vi "MS Auto Operation Demo.vi"() -> ()   [LabVIEW 2016]
uses:
  <vilib>/rvi/interface/nirviReadWriteControl/nirviReadWriteControl.xnode
  <vilib>/rvi/interface/nirviCloseFPGA/nirviCloseFPGA.xnode
  <vilib>/rvi/interface/nirviMethod/nirviMethod.xnode
  Subsystems/Global Variables.vi
  IRISS_FPGA_IO.vi
  <vilib>/Analysis/Matrix/Datatypes/RealMatrix.ctl
  <vilib>/Analysis/Matrix/NI_Matrix.lvlib
  Library/mjglib/var_OCTzHomeDir.vi
  Functions/EyeRobotDLL.dll
  FPGA Bitfiles/PhantomControlPI_FPGATarget_QuadCtr2_E2412E44.lvbitx
  Library/KevinLibraryAll/labview2011/kevLib2011.lvlib
  <vilib>/Math Plots/3D Math Plots/3D Scatter/3D Scatter Datatype/3D Scatter Datatype.lvclass
  <vilib>/Math Plots/3D Math Plots/3D Scatter/3D Scatter Datatype/Public/Plot Helper (Vector).vi
  <vilib>/platform/TimedLoop/XDataNode/XDataNode.xnode
  <vilib>/Platform/TimedLoop/XDataNode/nitl_modes.ctl
  <vilib>/Platform/TimedLoop/XDataNode/XDNodeRunTimeDep.lvlib
  <vilib>/Platform/TimedLoop/XDataNode/wakeup.ctl
  <vilib>/Platform/TimedLoop/XDataNode/timing_clust.ctl
  <vilib>/rvi/interface/nirviOpenFPGA/nirviOpenFPGA.xnode
  <vilib>/Utility/file.llb/Write Delimited Spreadsheet (string).vi
  <vilib>/Utility/file.llb/Write Delimited Spreadsheet (DBL).vi
  NiFpgaLv.dll
  <vilib>/Utility/error.llb/Error Cluster From Error Code.vi
  <vilib>/rvi/errors/niLvFpgaAdjustHostInterfaceError.vi
  <vilib>/FPGAPlugInAG/PXI-7833R/niLvFpga_Close_PXI-7833R.vi
  <vilib>/FPGAPlugInAG/PXI-7833R/niLvFpga_Open_PXI-7833R.vi
  <vilib>/FPGAPlugInAG/PXI-7833R/niLvFpga_Reset_PXI-7833R.vi
  <vilib>/Math Plots/3D Math Plots/3D Scatter/3D Scatter XCtrl/3D Scatter.xctl
panel:
  out "deltaRoll":sgl
  out "deltaXYZ":sgl[](array[numeric])
  out "Online Eye Model":T1
  in  "To Regulation":bool
  out "Trajectory Cluster":T2
  out "Eye Model Cluster":T4={"X Grid"=[], "Y Grid"=[], "Za_true Surf"=[], "Iris Center"=[], "Zp_true Surf"=[], "Pinv"=[[1.0, 0.0], [0.0, 1.0]], "za_true"=5.0, "za_work"=1.0, "zp_work"=-1.0, "zp_true"=-5.0}
  out "Update Mdl & Traj":bool=TRUE
  in  "Initialize":bool caption="To M/S"
  in  "Stage PID Cluster":T5={"Stage Z PID"={"Kp"=0.0005, "Kd"=0.001, "Ki"=0.0}, "Stage Y PID"={"Kp"=0.0003, "Kd"=0.01, "Ki"=0.0}, "Stage X PID"={"Kp"=0.0003, "Kd"=0.01, "Ki"=0.0}}
  in  "L1 to L4 PID Cluster":T6={"L1 PID Gains"={"Kp"=0.005, "Kd"=0.5, "Ki"=0.0005}, "L2 PID Gains"={"Kp"=0.01, "Kd"=1.0, "Ki"=0.0005}, "L3 PID Gains"={"Kp"=0.05, "Kd"=1.0, "Ki"=0.0005}, "L4 PID Gains"={"Kp"=0.1, "Kd"=1.0, "Ki"=0.0005}}
  in  "IRISS GUI":T7(tab)
  in  "Red Round Box":u32(colorbox)=16711690
  in  "Blue Round Box":u32(colorbox)=16860
  in  "Black Round Box":u32(colorbox)
  out "Vacuum Force [mmHg]  2":i32 caption="[mmHg]"
  in  "Vac Cmd [mmHg]":sgl min=0 max=600 step=50
  in  "IV Height [mmHg]":dbl=30.0 min=0.0 max=90.0 step=10.0
  in  "Irrigation":bool
  in  "Reroute Hold [sec]":dbl=10.0 caption="Hold [sec]"
  out "Next Speed":dbl=0.8 format="%#.2gx"
  out "Current Speed":dbl=0.2 format="%#_2gx"
  out "Next Depth":dbl=40.0 format="%#_g%%"
  out "Current Depth":dbl=20.0 format="%#_6g%%"
  in  "Depth Offset":dbl min=-30.0 max=70.0 step=5.0 format="%#_g%%"
  in  "Refractive Index":dbl=1.35
  in  "PO No-Fly":dbl=5.0 step=0.1 format="%#.2g"
  out "PO Cruising":dbl=5.0 format="%#.2g"
  in  "Iris Center":dbl=5.0 step=0.1 format="%#.2g"
  in  "AN Cruising":dbl=5.0 step=0.1 format="%#.2g"
  in  "AN No-Fly":dbl=5.0 step=0.1 format="%#.2g"
  in  "Iris XY Scaling":dbl[](array[numeric])=[1.0, 1.0] caption="Iris Scaling" min=0.5 max=2.0 step=0.05
  in  "Iris XY Center":dbl[](array[numeric])=[0.0, 5.0] caption="Iris Center" min=-5.0 max=5.0 step=0.25
  out "Asgn Pt Out of Bound":bool caption="Assign Pt OOB"
  out "Emergency alarm":bool
  out "Remote sender engaged":bool
  out "State changing":bool
  out "Current Run No.":u8
  out "No. of Runs":i32=5
  out "Tip out Posit":dbl[](array[numeric]) caption="Position [mm]" format="%#.3f"
  out "Tip cmd Posit":dbl[](array[numeric]) caption="Command [mm]" format="%#.3f"
  out "State Flag Array":bool[](array[boolean])
  in  "Speed Override":u16=3
  out "Timer":i32 format="%<%M:%S>t"
  in  "Assign Point [mm]":dbl[](array[numeric])=[0.0, -7.0, -6.0]
  in  "Go to Assign Pt":bool
  out "Irrigation Engaged?":bool caption="Irrigation Engaged"
  out "Robot XYZ":refnum<class "3D Plot Datatype.lvclass">[](xcontrol)
  in  "Offset":dbl[](array[numeric])
  in  "Radial Scale":dbl=0.5
  in  "Pattern":T8(ring)=enum."Centered"
  in  "Stop-and-Go":bool
  in  "SCAN_NO":string
  in  "Gen Traj":bool
  out "Trajectory OOB":bool
  out "Current System State":T9(ring)
  in  "Stage Z [mm]":dbl=100.0 min=-120.0 max=120.0 step=0.5
  in  "Stage Y [mm]":dbl=70.0 min=-120.0 max=100.0 step=0.5
  in  "Gripper":dbl
  in  "OCT Cmd Z [mm]":dbl min=-25.0 max=14.0 step=0.5
  out "Joint Out":dbl[](array[numeric])
  in  "XYZ Stage Power":bool
  in  "Arm Power":bool
  out "Robot Status Array":bool[](array[boolean])
  in  "L1 [deg]":dbl=-40.0
  in  "L2 [deg]":dbl=15.0
  in  "L3 [mm]":dbl=-5.0 step=0.1
  out "Status 2":bool[](array[boolean])
  in  "L4 [deg]":dbl=-10.0 step=0.1
  in  "Home":bool
  out "OCT Z out [mm]":dbl caption="OCT Out Z [mm]" format="%#.4f"
  in  "Tool Type":i32=6
  in  "Tool Offset [mm]":dbl=-50.68
  out "Grasp out":dbl format="%#.2g"
  in  "OCTz Home Dir":bool
  in  "OCT Z PID Gains":cluster{"Kp":dbl, "Kd":dbl, "Ki":dbl}={"Kp"=0.0003, "Kd"=0.0001, "Ki"=0.01}
  in  "Remote Control Source":u16(ring) caption="Remote Source" items=["None", "Surgical Console", "Joystick", "MJG Teleoperation", "MJG C++ Teleoperation"]
  in  "Reset Joystick":bool caption="Encoder Reset"
  out "Send Count":u64
  out "Receive Count":u64
  out "Arm ID":i32
  out "Status":bool
  in  "Stage X [mm]":dbl=30.0 min=-120.0 max=120.0 step=0.5
  out "XYZ Stage Out":dbl[](array[numeric])
  in  "Use Online Scan":bool
  out "Z Stage cmd [mm]":dbl=6.0 caption="Reference Z [mm]" min=0.0 max=12.0 step=0.5
  out "Y Stage cmd [mm]":dbl=6.0 caption="Reference Y  [mm]" min=0.0 max=12.0 step=0.5
  out "X Stage cmd [mm]":dbl=6.0 caption="Reference X [mm]" min=0.0 max=12.0 step=0.5
  in  "Process VSCAN":bool
  in  "Restart":bool
  out "Generation Error":errorcluster
  out "Model Created":bool
  out "Pressure Plots":T10(graph)
  in  "Eye No":i16=1 min=1 step=1
  in  "Reroute Transit Vacf":dbl=100.0
  in  "Z Rot Axis":dbl=1.0
  in  "Z Dist Thld":dbl[](array[numeric])=[3.0, 5.0] caption="Z Distance Threshould"
  in  "Vac Extremum":dbl[](array[numeric])=[68.0, 68.0] caption="Vacuum Extremum"
  in  "Max Limit [mmHg]":dbl=600.0 min=0.0 max=600.0 step=100.0
  out "Value [mmHg]":i8
  in  "Target IOP":sgl=20.0 min=0 max=100 step=1 format="%#_13g"
  in  "PID ON/OFF":bool
  in  "Hydration":bool
  in  "IOP PID Gains":cluster{"Kp":dbl, "Kd":dbl, "Ki":dbl, "Ts":dbl}={"Kp"=5.0, "Kd"=0.0, "Ki"=5.0, "Ts"=0.01}
  in  "Save Data":bool
  out "File Exists":bool
  out "File Path":path
  out "Elaspsed Time [s]":sgl
  in  "Data No":i16=1 min=1 step=1
  out "Pressure Reading":dbl[](array[numeric]) caption="IOP Output [mmHg]"
  in  "Total Time":i16=90 min=1 step=1
  in  "Min PC Gap":dbl=0.1 caption="Min PC Gap [mm]" min=0.0 max=10.0 step=0.1 format="%#.3g"
  in  "Min AC Gap":dbl=0.1 caption="Min AC Gap [mm]" min=0.0 max=10.0 step=0.1 format="%#.3g"
  out "Scaling":dbl[](array[numeric])=[1.0, 1.0, 1.0] caption="S" min=0.5 max=1.5 step=0.05 format="%#_3g"
  in  "Joint Limits":dbl[][](array[numeric])=[[-68.0, -4.0], [-26.0, 52.0], [-40.0, 23.0], [-180.0, 180.0]] format="%#.3g"
  out "First Trk Pt":dbl[](array[numeric]) format="%#.3g"
  out "Error(s) Out on Program End":errorcluster
  out "L4 Waveform Graph":dbl[](graph)
  out "L3 Waveform Graph":dbl[](graph)
  out "L2 Waveform Graph":dbl[](graph)
  out "L1 Waveform Graph":dbl[](graph)
  in  "Aiming Pt":dbl[](array[numeric])=[-40.0, 11.0, 2.0, 0.0] format="%#.3g"
  in  "Engage Pt":dbl[](array[numeric])=[-40.0, 11.0, 2.0, 0.0] format="%#.3g"
  in  "Rotation":dbl[](array[numeric])=[0.0, 0.0, 0.0] caption="R [deg]" min=-15.0 max=15.0 step=0.5 format="%#_3g"
  out "Translation":dbl[](array[numeric]) caption="T [mm]" min=-3.0 max=3.0 step=0.1 format="%#_3g"
  in  "Inc Ctrl":dbl[](array[numeric])=[0.1, 0.05, 0.05] caption="Increment Control"
  in  "Depth Ctrl Array\n(% Thickness)":dbl[](array[numeric])=[40.0, 60.0, 80.0] min=10.0 max=90.0 step=5.0 format="%#_g%%"
  in  "Load Traj":bool caption="To M/S"
  in  "MS/Auto":bool
  in  "Retract":bool caption="To M/S"
  in  "Stop Accurus":bool caption="To M/S"
  in  "L3 Go Home":bool caption="To M/S"
  in  "Track":bool caption="To M/S"
  in  "Insert":bool caption="To M/S"
  in  "Program Stop":bool
  # "M/S\n\nAuto"
  # "Tool Tip Location"
  # "Tracking Planning"
  # "RCM"
  # "X\nY\nZ"
  # "X\nY\nZ"
  # "Tool"
  # "Trajectory"
  # "System Progress"
  # "Assign Point Rerouting"
  # "Trajectory Generation"
  # "X\nY\nZ"
  # "X Offset"
  # "Y Offset"
  # "Homing finished"
  # "Z Offset"
  # "M/S initialization finished"
  # "Tool Cruising Boundaries"
  # "XY-plane"
  # "Trajecoty loading finished"
  # "Aiming finished"
  # "Tool engaged"
  # "Z-axis"
  # "Tracking initialization finished"
  # "In Tracking"
  # "Bausch Lomb"
  # "Rerouting finished"
  # "X\nY"
  # "X\nY"
  # "In regulation"
  # "Homing"
  # "Robot Control"
  # "Joint Definition"
  # "Arm"
  # "Tool"
  # "Stage"
  # "Joint M/S Cmd"
  # "Robot Status"
  # "ROBOT_HARDWARE_NOT_PRESENT"
  # "ROBOT_HARDWARE_NOT_FOUND_ALL_DRIVES"
  # "ROBOT_HARDWARE_SENSOR_FAULT"
  # "ROBOT_NOT_RUNNING"
  # "ROBOT_COMMUNICATION_ERROR"
  # "OCT Control"
  # "ROBOT_KINEMATICS_NO_SOLUTION"
  # "ROBOT_KINEMATICS_INSERTION_LENGTH_TOO_SMALL"
  # "ROBOT_COMMAND_BEYOND_JOINT_RANGE"
  # "ROBOT_COMMAND_TOO_LARGE"
  # "XYZ Stage Control"
  # "Eye Model Creation"
  # "Irrigation and Aspiration"
  # "IOP Control"
  # "Data Saving"
  # "Irrigation"
  # "Aspiration"
  # "ACh"
  # "Vitreous"
  # "Rotation & Vacuum Force Scheduling"
  # "Joint Motion & Control"
  # "Space Deform Parameters"
  # "Depth Ctrl"
  # "S"
  # "R"
  # "[deg]"
  # "T"
  # "[mm]"
  # "First Track Point"
  # "AC & PC Gap"
  # "X1"
  # "[mm]"
  # "Y"
  # "[mm]"
  # "Z"
  # "[mm]"
  # "L4"
  # "[deg]"
  # "Joint Limits"
  # "Error Message"
  # "Incision"
  # "Min."
  # "Max."
  # "L1"
  # "[deg]"
  # "L1"
  # "L2"
  # "L2"
  # "[deg]"
  # "L3"
  # "[mm]"
  # "L3"
  # "L4"
  # "[deg]"
  # "L4"
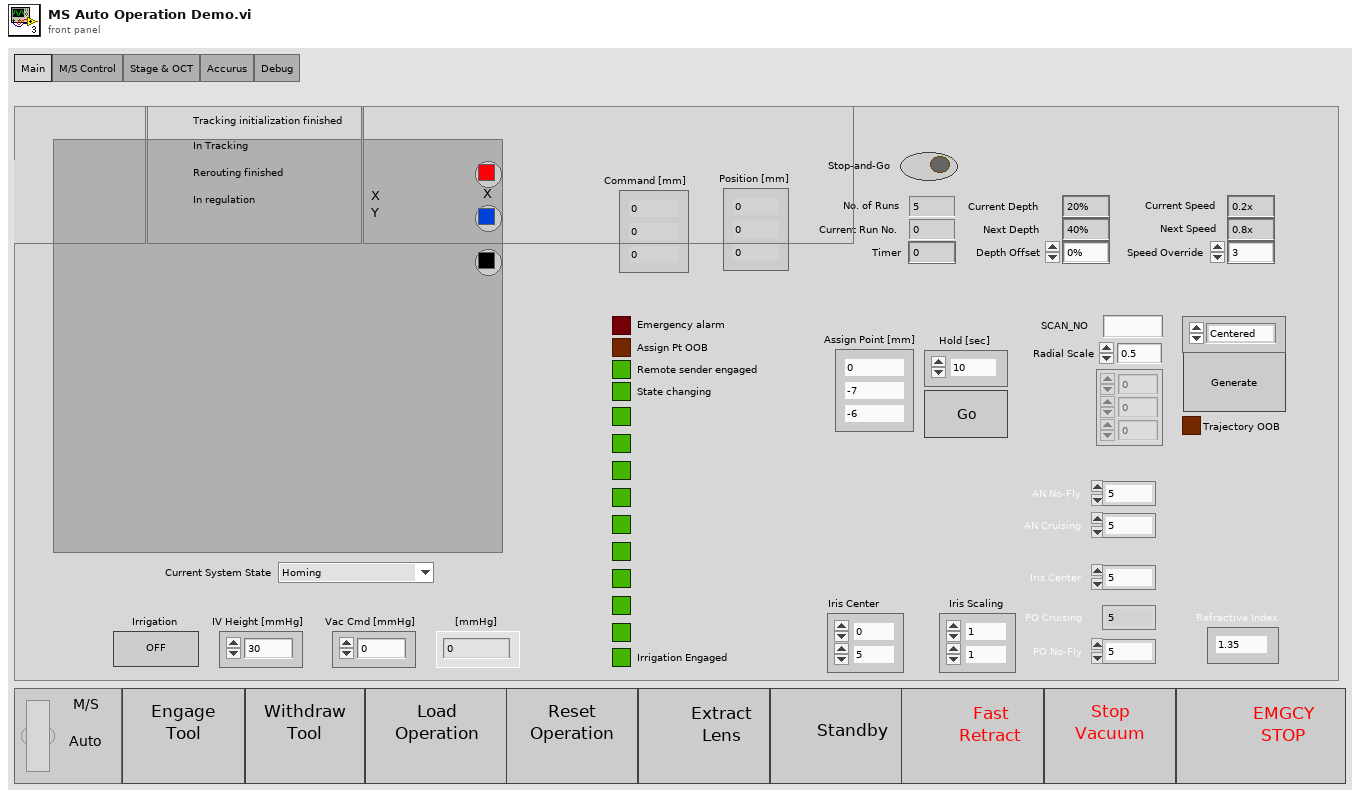
[diagram p1: front panel]
types:
  T1 = cluster{"za_true":dbl, "za_work":dbl, "zi":dbl, "zp_work":dbl, "zp_true":dbl, "Iris XY Center":dbl[], "Iris XY Scaling":dbl[]}
  T2 = cluster{"Traj Px Array":dbl[], "Traj Py Array":dbl[], "Traj Pz Array":dbl[], "Speed Array":dbl[], "Depth Array":dbl[]}
  T3 = typedef "NI_Matrix.lvlib/RealMatrix.ctl" = dbl[][]
  T4 = cluster{"X Grid":dbl[], "Y Grid":dbl[], "Za_true Surf":dbl[][], "Iris Center":dbl[], "Zp_true Surf":dbl[][], "Pinv":T3, "za_true":dbl, "za_work":dbl, "zp_work":dbl, "zp_true":dbl}
  T5 = cluster{"Stage Z PID":cluster{"Kp":dbl, "Kd":dbl, "Ki":dbl}, "Stage Y PID":cluster{"Kp":dbl, "Kd":dbl, "Ki":dbl}, "Stage X PID":cluster{"Kp":dbl, "Kd":dbl, "Ki":dbl}}
  T6 = cluster{"L1 PID Gains":cluster{"Kp":dbl, "Kd":dbl, "Ki":dbl}, "L2 PID Gains":cluster{"Kp":dbl, "Kd":dbl, "Ki":dbl}, "L3 PID Gains":cluster{"Kp":dbl, "Kd":dbl, "Ki":dbl}, "L4 PID Gains":cluster{"Kp":dbl, "Kd":dbl, "Ki":dbl}}
  T7 = enum32{"Main", "M/S Control", "Stage & OCT", "Accurus", "Debug"}
  T8 = enum16{"Entry Site", "Centered", "Insertion", "Extraction", "Reverse Entry Site", "Reverse Centered"}
  T9 = enum16{"Homing", "M/S Initialization", "M/S Operation", "Aiming", "Engaging", "Trajectory Loading", "Tracking Initialization", "Tracking", "Rerouting", "Regulation"}
  T10 = cluster{"Pressure Reading[0]":dbl, "Pressure Reading[1]":dbl, "Pressure Reading[2]":dbl, "Pressure Reading[3]":dbl, "Pressure Reading[4]":dbl, "Pressure Reading[5]":dbl, "Pressure Reading[6]":dbl, "Pressure Reading[7]":dbl, "Pressure Reading[8]":dbl}
  T11 = cluster{"Prev L1 to L4 Posit":dbl[], "Prev Stage Posit":dbl[], "Prev OCT Z Posit":dbl}
  T12 = typedef "XDNodeRunTimeDep.lvlib/timing_clust.ctl" = cluster{"Expected End [f-1]":u64, "Actual End [f-1]":u64, "Finished Late? [f-1]":bool, "Expected End [i-1]":u64, "Actual End [i-1]":u64, "Finished Late? [i-1]":bool, "Expected Start [i]":u64, "Actual Start [i]":u64, "Expected Start [f]":u64, "Actual Start [f]":u64, "Source Name":string, "Structure Name":string, "Period":i64, "Deadline":i64, "Offset":i64, "Start":i64, "Priority":i32, "Timeout":i32, "Mode":T13, "Wakeup Reason":T14, "Error":errorcluster, "Source Type":string, "Secondary Source Type":string, "Global End Time":u64, "Global Start Time":u64, "Frame Duration":u64, "Iteration Duration":u64, "Assigned CPU":i32, "I/O Scan Engine Mode":u32}
  T13 = typedef "XDNodeRunTimeDep.lvlib/nitl_modes.ctl" = enum32{"No Change", "Process missed periods, maintain original phase", "Discard missed periods, maintain original phase", "Process missed periods, ignore original phase", "Discard missed periods, ignore original phase"}
  T14 = typedef "XDNodeRunTimeDep.lvlib/wakeup.ctl" = enum32{"Normal", "Aborted", "Asynchronous wakeup", "Timing source error", "Timed loop error", "Timeout"}
  T15 = cluster{"L1 to L4 PID Cluster":cluster{"L1 PID Gains":cluster{"Kp":dbl, "Kd":dbl, "Ki":dbl}, "L2 PID Gains":cluster{"Kp":dbl, "Kd":dbl, "Ki":dbl}, "L3 PID Gains":cluster{"Kp":dbl, "Kd":dbl, "Ki":dbl}, "L4 PID Gains":cluster{"Kp":dbl, "Kd":dbl, "Ki":dbl}}, "Stage PID Cluster":cluster{"Stage Z PID":cluster{"Kp":dbl, "Kd":dbl, "Ki":dbl}, "Stage Y PID":cluster{"Kp":dbl, "Kd":dbl, "Ki":dbl}, "Stage X PID":cluster{"Kp":dbl, "Kd":dbl, "Ki":dbl}}, "OCT Z PID Gains":cluster{"Kp":dbl, "Kd":dbl, "Ki":dbl}}
  T16 = enum8{"Enabled", "Disabled", "Disabled and Grayed Out"}
  T17 = cluster{"IOP Output [mmHg][0]":dbl, "IOP Output [mmHg][1]":dbl, "IOP Output [mmHg][2]":dbl, "IOP Output [mmHg][3]":dbl, "IOP Output [mmHg][4]":dbl, "IOP Output [mmHg][5]":dbl, "IOP Output [mmHg][6]":dbl, "IOP Output [mmHg][7]":dbl, "IOP Output [mmHg][8]":dbl}
  T18 = cluster{"Last L1 to L4 Posit":dbl[], "Last Stage Posit":dbl[], "Last OCT Z Posit":dbl}
  T19 = cluster{"za_true_0":dbl, "za_work_0":dbl, "zp_work_0":dbl, "zp_true_0":dbl, "IrisCenter_0":dbl[]}
  T20 = cluster{"X Grid":dbl[], "Y Grid":dbl[], "Za_true Surf":dbl[][], "Iris Center":dbl[], "Zp_true Surf":dbl[][], "Real Matrix":T3, "za_true":dbl, "za_work":dbl, "zp_work":dbl, "zp_true":dbl}
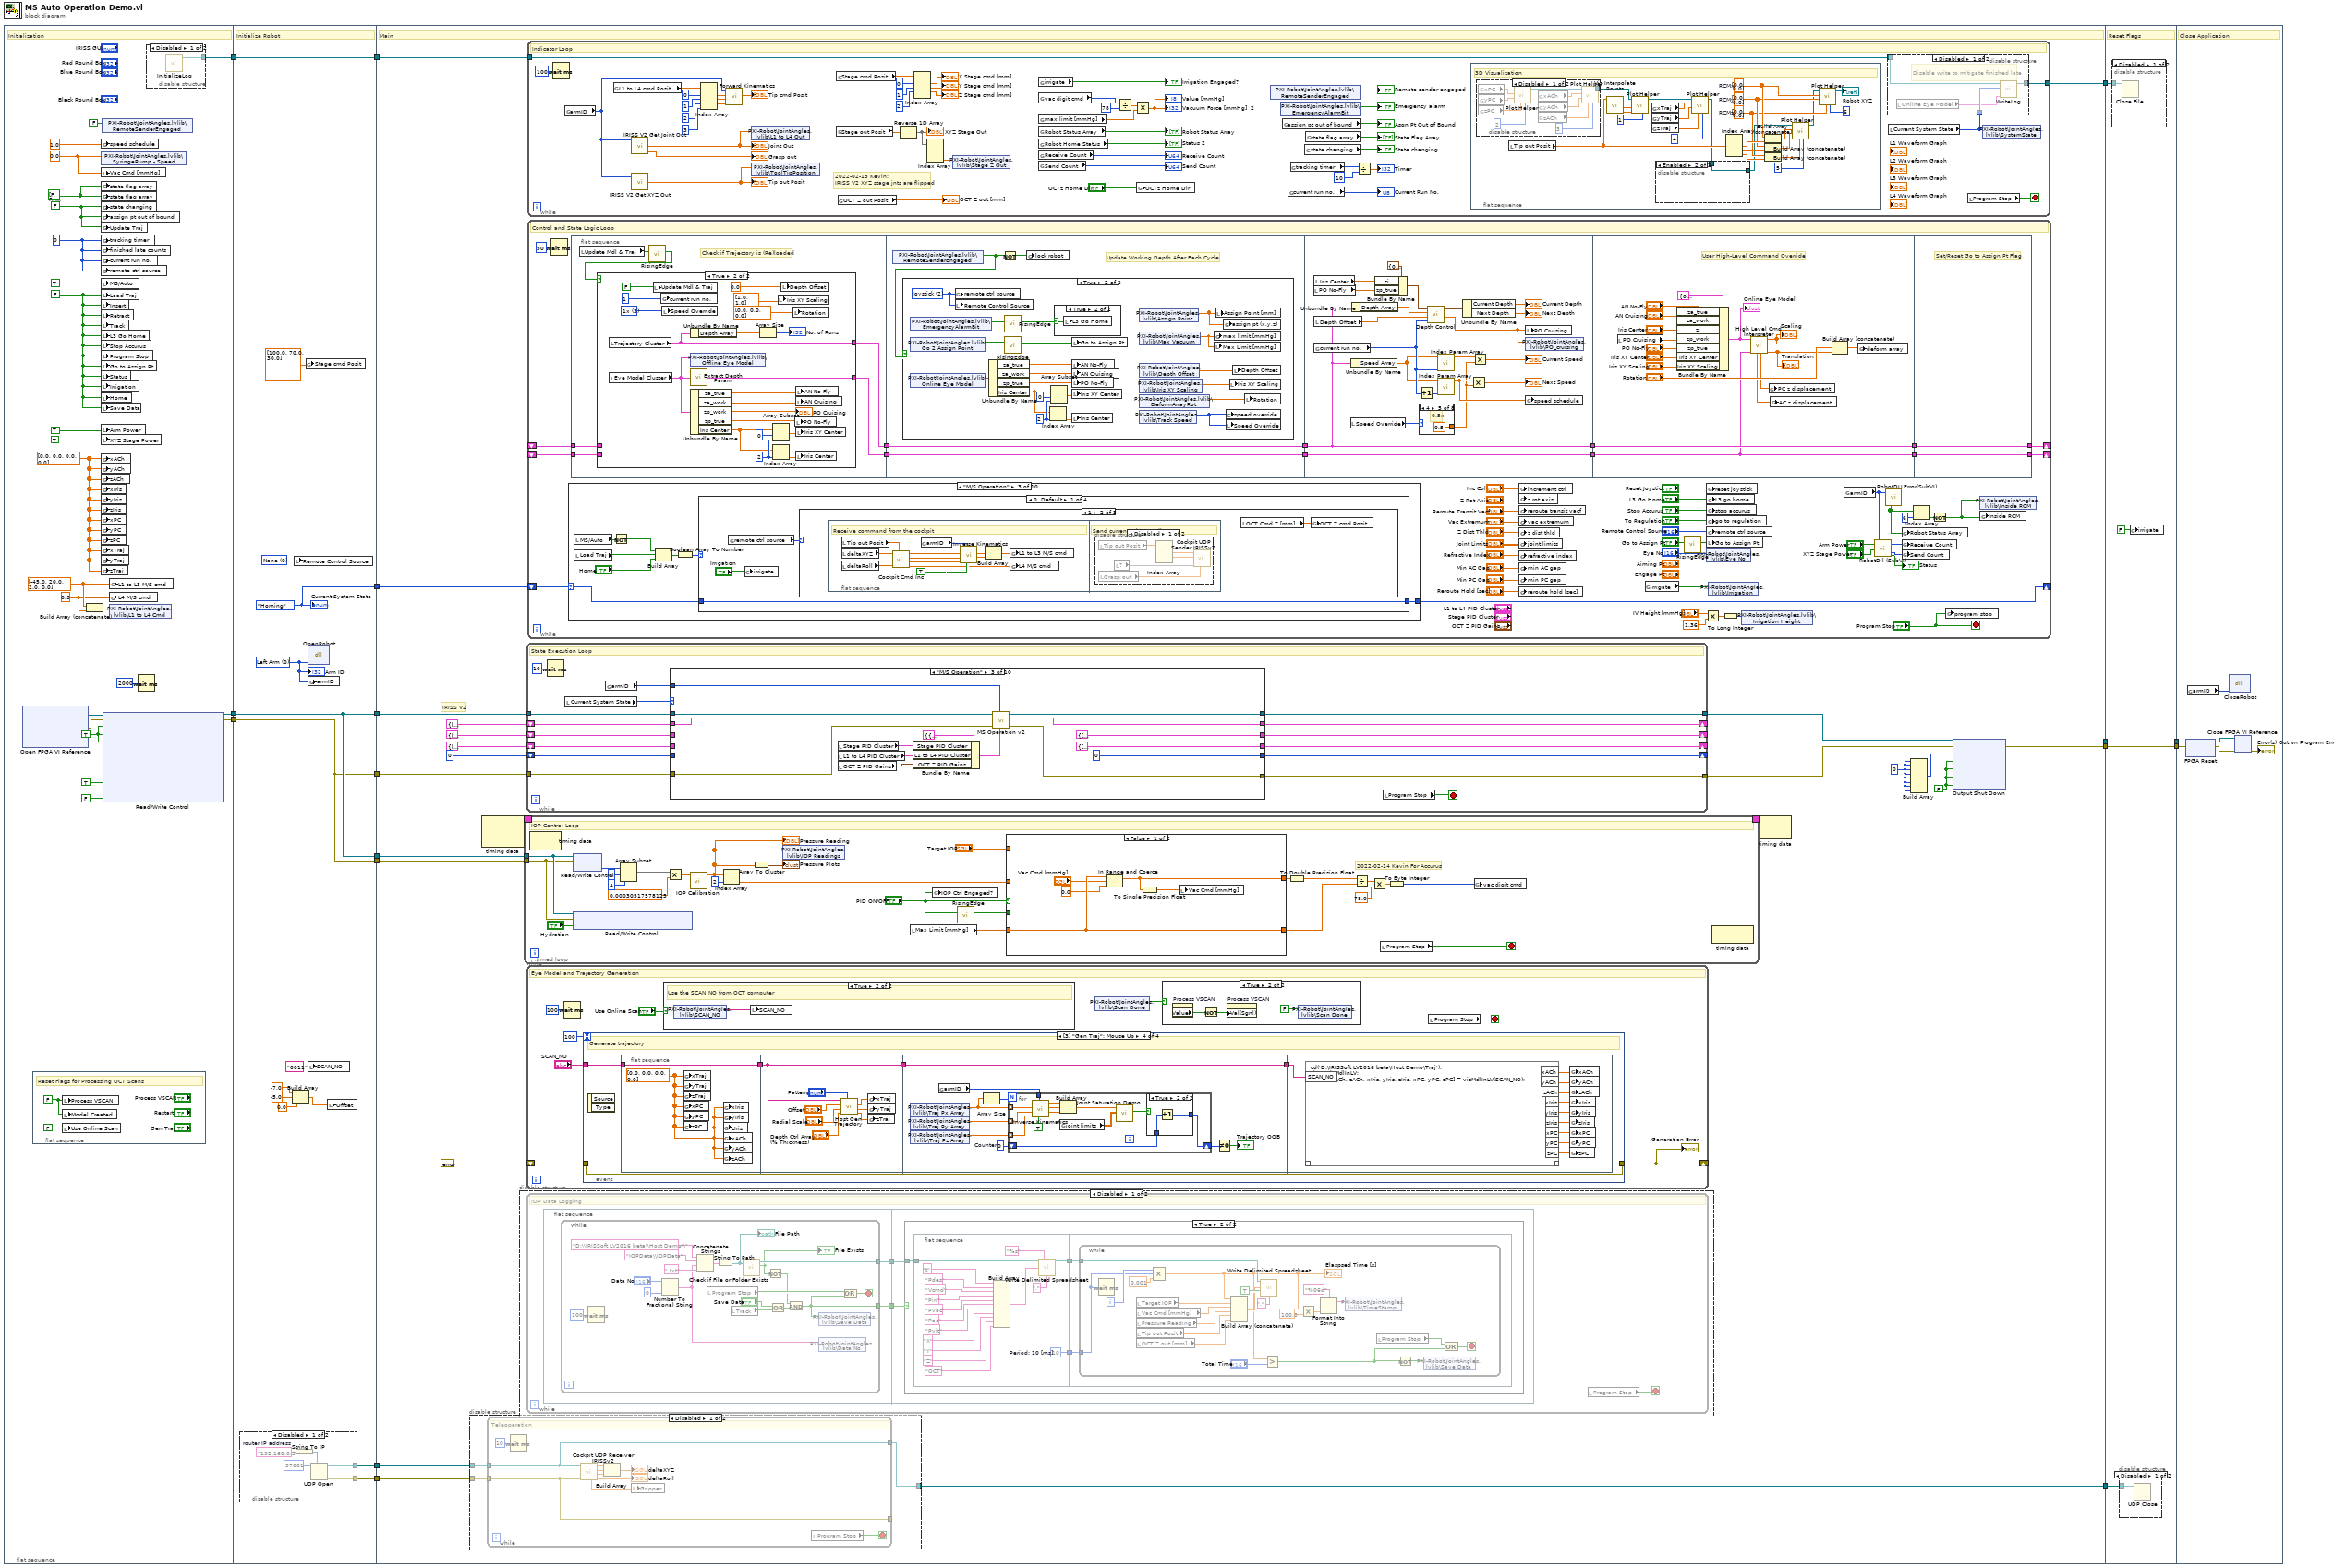
[diagram p0: block diagram]
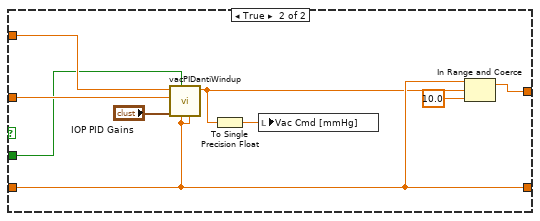
[diagram p7: hidden frame]
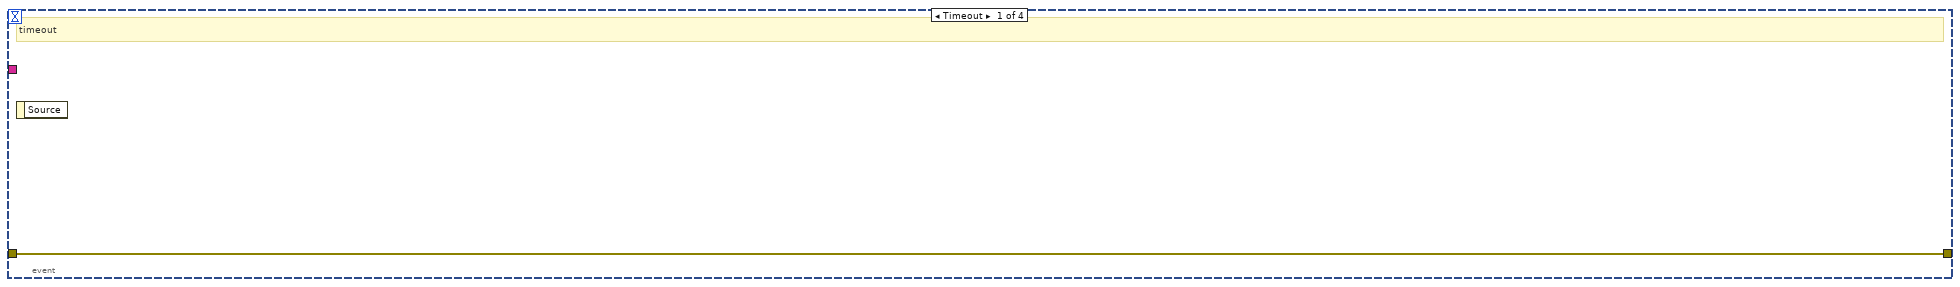
[diagram p10: hidden frame]
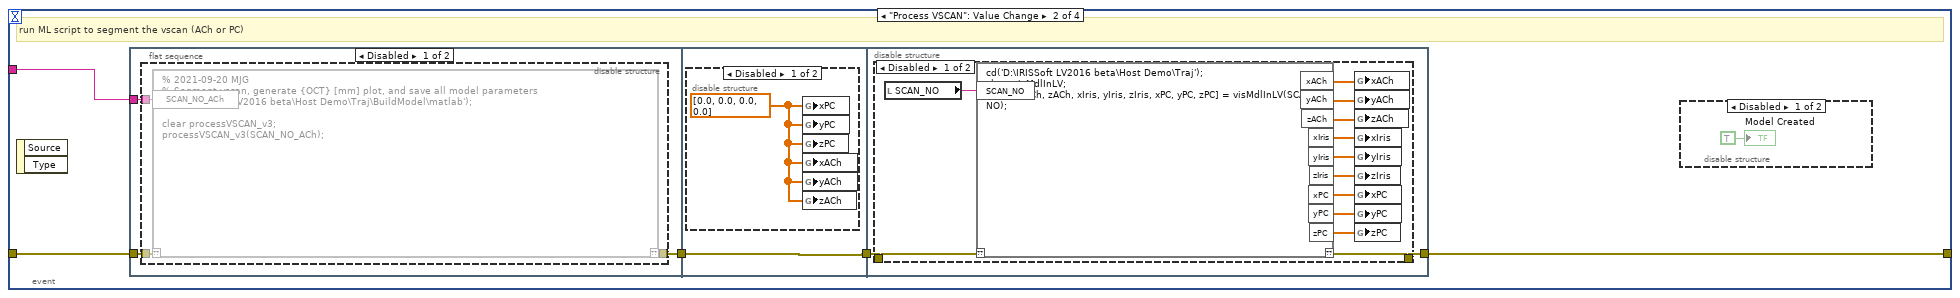
[diagram p11: hidden frame]
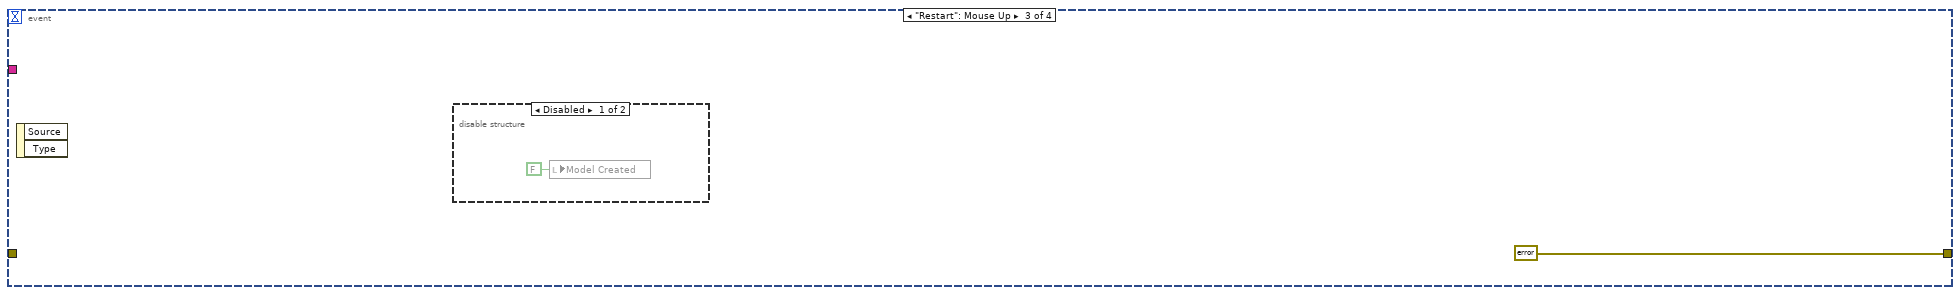
[diagram p16: hidden frame]
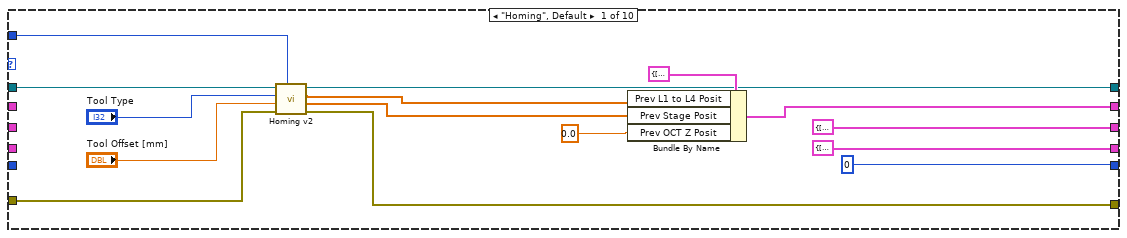
[diagram p19: hidden frame]
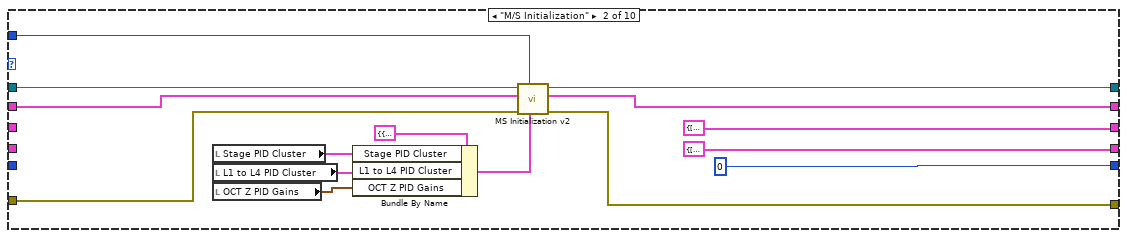
[diagram p20: hidden frame]
diagram:
  n1 = flat-sequence {
    tunnel: [w39] -> w9
    tunnel: [w27] -> w5
    tunnel: [w26] -> w4
    tunnel: [w54] -> w12
    tunnel: [w55] -> w11
    tunnel: [w53] -> w10
    tunnel: w9 -> [w57]
    tunnel: [w57] -> w8
    tunnel: [w55] -> w7
    tunnel: [w54] -> w6
    tunnel: w5 -> [w55]
    tunnel: w4 -> [w54]
    tunnel: [w52] -> w3
    tunnel: [w51] -> w2
    tunnel: w12 -> [w83]
    tunnel: w11 -> [w80]
    tunnel: w10 -> [w86]
    tunnel: [w81] -> w17
    tunnel: [w82] -> w16
    tunnel: w8 -> [w85]
    tunnel: [w84] -> w15
    tunnel: w7 -> [w70]
    tunnel: w6 -> [w69]
    tunnel: w3 -> [w65]
    tunnel: w2 -> [w64]
    tunnel: [w63] -> w1
    tunnel: w17 -> [w1060]
    tunnel: w16 -> [w1061]
    tunnel: w15 -> [w1062]
    tunnel: [w1061] -> w14
    tunnel: [w1060] -> w13
    tunnel: w1 -> [w1058]
    tunnel: w14 -> [w1070]
    tunnel: w13 -> [w1069]
    frame #0 {
      w28 = TRUE ("Conn0/DIO13 Button 2")
      w24 = dbl[] [0.0, 0.0, 0.0, 0.0] ("First Trk Pt 2")
      w34 = 0.0 ("L4 M/S cmd")
      w35 = dbl[] [-45.0, 20.0, 2.0, 0.0] ("First Trk Pt 2")
      w38 = 0.0 ("SyringePump - Speed")
      w23 = 0 ("finished late counts")
      w37 = bool[] [FALSE, FALSE, FALSE, FALSE, FALSE, FALSE, FALSE, FALSE, FALSE] ("state flag array")
      w32 = FALSE ("state changing")
      w25 = FALSE ("program stop")
      # "Initialization"
      n2 = xnode "Open FPGA VI Reference"() -> ("FPGA VI Reference Out"=w22:refnum<k20>, "error out"=w21:errorcluster)  [unwired: 2 in]
      n3 = flat-sequence {
        frame #0 {
          w41 = FALSE ("ACh Processed")
          # "Reset Flags for Processing OCT Scans"
          n4 = local write "Process VSCAN"(w41) -> ()
          n5 = local write "Model Created"(w41) -> ()
          n6 = local write "Use Online Scan"(FALSE ("Use Online Scan")) -> ()
        }
      }
      n7 = Build Array (concatenate)(w35, w34) -> (w33:dbl[])
      n8 = global write "Global Variables.vi" "speed schedule"(1.0 ("speed schedule")) -> ()
      n9 = shared-variable "PXI-Robot\\JointAngles.lvlib\\SyringePump - Speed"(w38) -> ()  [unwired: 1 in, 1 out]
      n10 = local write "Vac Cmd [mmHg]"(w38) -> ()
      n11 = global write "Global Variables.vi" "state flag array"(w37) -> ()
      n12 = global write "Global Variables.vi" "state flag array"(w37) -> ()
      n13 = global write "Global Variables.vi" "state changing"(w32) -> ()
      n14 = global write "Global Variables.vi" "assign pt out of bound"(w32) -> ()
      n15 = global write "Global Variables.vi" "Update Traj"(w32) -> ()
      n16 = global write "Global Variables.vi" "tracking timer"(w23) -> ()
      n17 = global write "Global Variables.vi" "finished late counts"(w23) -> ()
      n18 = global write "Global Variables.vi" "current run no."(w23) -> ()
      n19 = global write "Global Variables.vi" "remote ctrl source"(w23) -> ()
      n20 = local write "MS/Auto"(TRUE ("MS/Auto")) -> ()
      n21 = local write "Load Traj"(w25) -> ()
      n22 = local write "Insert"(w25) -> ()
      n23 = local write "Retract"(w25) -> ()
      n24 = local write "Track"(w25) -> ()
      n25 = local write "L3 Go Home"(w25) -> ()
      n26 = local write "Stop Accurus"(w25) -> ()
      n27 = local write "Program Stop"(w25) -> ()
      n28 = local write "Go to Assign Pt"(w25) -> ()
      n29 = local write "Status"(w25) -> ()
      n30 = local write "Irrigation"(w25) -> ()
      n31 = local write "Home"(w25) -> ()
      n32 = local write "Save Data"(w25) -> ()
      n33 = local write "Arm Power"(TRUE ("Arm ON/OFF")) -> ()
      n34 = local write "XYZ Stage Power"(TRUE ("Arm ON/OFF")) -> ()
      n35 = global write "Global Variables.vi" "xACh"(w24) -> ()
      n36 = global write "Global Variables.vi" "yACh"(w24) -> ()
      n37 = global write "Global Variables.vi" "zACh"(w24) -> ()
      n38 = global write "Global Variables.vi" "xIris"(w24) -> ()
      n39 = global write "Global Variables.vi" "yIris"(w24) -> ()
      n40 = global write "Global Variables.vi" "zIris"(w24) -> ()
      n41 = global write "Global Variables.vi" "xPC"(w24) -> ()
      n42 = global write "Global Variables.vi" "yPC"(w24) -> ()
      n43 = global write "Global Variables.vi" "zPC"(w24) -> ()
      n44 = global write "Global Variables.vi" "xTraj"(w24) -> ()
      n45 = global write "Global Variables.vi" "yTraj"(w24) -> ()
      n46 = global write "Global Variables.vi" "zTraj"(w24) -> ()
      n47 = shared-variable "PXI-Robot\\JointAngles.lvlib\\RemoteSenderEngaged"(FALSE ("RemoteSenderEngaged")) -> ()  [unwired: 1 in, 1 out]
      n48 = xnode "Read/Write Control"("FPGA VI Reference In"=w22, "error in"=w21, "Conn0/DIO12 Button 1"=w28, "Conn0/DIO13 Button 2"=w28, "Conn0/DIO15 Button 4"=w28, "Reset 14"=TRUE, "Hydration On/Off (Connector2/DIO28)"=FALSE) -> ("FPGA VI Reference Out"=w27:refnum<k20>, "error out"=w26:errorcluster)  [unwired: 3 in, 2 out]
      n49 = global write "Global Variables.vi" "L1 to L3 M/S cmd"(w35) -> ()
      n50 = global write "Global Variables.vi" "L4 M/S cmd"(w34) -> ()
      n51 = shared-variable "PXI-Robot\\JointAngles.lvlib\\L1 to L4 Cmd"(w33) -> ()  [unwired: 1 in, 1 out]
      n52 = Wait (ms)(milliseconds to wait=u32 2000) -> ()  [unwired: 1 out]
      n53 = disable-structure shown="Disabled" {
        disable-tunnel: [w43 _] -> w39
        frame Disabled {
          n54 = call "InitializeLog.vi"() -> ("Byte Stream File out"=w43:refnum<file>)  [unwired: 11 in]
        }
        frame Enabled {
        }
      }
    }
    frame #1 {
      w49 = u16 0 items=["None", "Surgical Console", "Joystick", "MJG Teleoperation", "MJG C++ Teleoperation"] ("Remote Control Source 2")
      w53 = T9."Homing" ("Current State")
      w56 = 0 items=["Left Arm", "Right Arm"] ("Left or Right Arm")
      # "Initialize Robot"
      n55 = disable-structure shown="Disabled" {
        disable-tunnel: [w59 _] -> w52
        disable-tunnel: [w58 _] -> w51
        frame Disabled {
          w61 = "192.168.0.3"  # router IP address
          n56 = String To IP(1:w61) -> (0:w60:u32)
          n57 = UDP Open(7:w60, 11:u16 37001 ("port")) -> (port=w59:refnum<k16>, 0:w58:errorcluster)  [unwired: 3 in, 1 out]
        }
        frame Enabled {
        }
      }
      n58 = Build Array(-7.0 ("element"), -5.0 ("element"), 0.0 ("element")) -> (w48:dbl[])
      n59 = local write "Remote Control Source"(w49) -> ()
      n60 = global write "Global Variables.vi" "Stage cmd Posit"(dbl[] [100.0, 70.0, 30.0] ("Stage cmd Posit")) -> ()
      n61 = dll-call lib="D:/Kevin/IRISS V2 dev/Host Demo/Functions/EyeRobotDLL.dll" fn="OpenRobot" label="Open"("id"=w56) -> ()  [unwired: 5 in, 2 out]
      n62 = global write "Global Variables.vi" "armID"(w56) -> ()
      n63 = local write "SCAN_NO"("0011" ("SCAN_NO")) -> ()
      n64 = local write "Offset"(w48) -> ()
      "Arm ID" <- w56
      "Current System State" <- w53
    }
    frame #2 {
      w68 = FALSE
      w66 = i16 0 ("element")
      # "IRISS V2"
      # "Main"
      n65 = disable-structure shown="Disabled" {
        disable-tunnel: w65 -> [w158 _]
        disable-tunnel: w64 -> [w157 _]
        disable-tunnel: [w156 _] -> w63
        frame Disabled {
          n66 = while {
            tunnel: w158 -> [w165]
            tunnel: w157 -> [w164]
            tunnel: [w165] -> w156
            tunnel: [w164] -> _
            stop <- w163 stop-if-true
            # "Teleoperation"
            n67 = Wait (ms)(milliseconds to wait=u32 10) -> ()  [unwired: 1 out]
            n68 = call "Cockpit UDP Receiver IRISSv2.vi"("error in"=w164, "port"=w165) -> ("deltaRoll"=→"deltaRoll":sgl, "deltaZ"=w166:sgl, "deltaY"=w167:sgl, "deltaX"=w168:sgl, "gripper"=w160:sgl)  [unwired: 5 in]
            n69 = Build Array(w168, w167, w166) -> (→"deltaXYZ":sgl[])
            n70 = local write "Gripper"(w160) -> ()
            n71 = local read "Program Stop"() -> (w163:bool)
          }
        }
        frame Enabled {
        }
      }
      n72 = node-c288() -> (w72:T12)  [unwired: 2 in]
      n73 = disable-structure shown="Disabled" {
        frame Disabled {
          n74 = while {
            stop <- w87 stop-if-true
            # "IOP Data Logging"
            n75 = flat-sequence {
              tunnel: [w90] -> w89
              tunnel: [w91] -> w88
              tunnel: w89 -> [w111]
              tunnel: w88 -> [w110]
              frame #0 {
                n76 = while {
                  tunnel: [w108] -> w91
                  tunnel: [w92] -> w90
                  stop <- w109 stop-if-true
                  n77 = Wait (ms)(milliseconds to wait=u32 100) -> ()  [unwired: 1 out]
                  n78 = Number To Fractional String(number="Data No", precision (6)=i16 0) -> (F-format string=w98:string)  [unwired: 2 in]
                  n79 = Concatenate Strings("D:\\IRISSoft LV2016 beta\\Host Demo\\", "IOPData\\IOPData", w98, ".txt" ("string")) -> (w104:string)
                  n80 = local read "Program Stop"() -> (w105:bool)
                  n81 = String To Path(string=w104) -> (path=w100:path)
                  "File Path" <- w100
                  n82 = local read "Track"() -> (w95:bool)
                  n83 = call <vilib>:"Check if File or Folder Exists.vi"("path"=w100) -> ("file or folder exists?"=w106:bool, "dup path"=w108:path)  [unwired: 8 in, 1 out]
                  "File Exists" <- w106
                  n84 = Not(x=w106) -> (.not. x?=w94:bool)
                  n85 = Or(x="Save Data", y=w95) -> (x .or. y?=w93:bool)
                  n86 = Compound Arithmetic op=AND(w94, w93) -> (w92:bool)
                  n87 = shared-variable "PXI-Robot\\JointAngles.lvlib\\Save Data"(w92) -> ()  [unwired: 1 in, 1 out]
                  n88 = shared-variable "PXI-Robot\\JointAngles.lvlib\\Data No"(w98) -> ()  [unwired: 1 in, 1 out]
                  n89 = Compound Arithmetic op=OR(w105, w92) -> (w109:bool)
                }
              }
              frame #1 {
                n90 = case shown="True" w111 {
                  tunnel: w110 -> [_ w114]
                  frame False {
                  }
                  frame True {
                    n91 = flat-sequence {
                      tunnel: w114 -> [w125]
                      tunnel: [w123] -> w113
                      tunnel: [w119] -> w112
                      tunnel: w113 -> [w133]
                      tunnel: w112 -> [w132]
                      frame #0 {
                        w119 = 10  # Period: 10 [ms]
                        n92 = Build Array("t" ("delimiter (\\t)"), "Pdes" ("delimiter (\\t)"), "Vcmd" ("delimiter (\\t)"), "Pirr" ("delimiter (\\t)"), "Pvac" ("delimiter (\\t)"), "Pac" ("delimiter (\\t)"), "Pvit" ("delimiter (\\t)"), "X" ("delimiter (\\t)"), "Y" ("delimiter (\\t)"), "Z" ("delimiter (\\t)"), "OCT" ("delimiter (\\t)")) -> (w122:string[])
                        n93 = call-poly <vilib>:"Write Delimited Spreadsheet.vi"("file path (dialog if empty)"=w125, "format (%s)"="%s", "1D data"=w122, "delimiter (\\t)"="," ("delimiter (\\t)")) -> ("new file path (Not A Path if cancelled)"=w123:path)  [unwired: 10 in, 1 out]
                      }
                      frame #1 {
                        n94 = while {
                          tunnel: w133 -> [w152]
                          tunnel: w132 -> [w138]
                          i -> [w153]
                          stop <- w155 stop-if-true
                          n95 = Wait (ms)(milliseconds to wait=w138) -> ()  [unwired: 1 out]
                          n96 = local read "Target IOP"() -> (w148:sgl)
                          n97 = local read "Vac Cmd [mmHg]"() -> (w147:sgl)
                          n98 = local read "Pressure Reading"() -> (w146:dbl[])
                          n99 = local read "Tip out Posit"() -> (w143:dbl[])
                          n100 = local read "OCT Z out [mm]"() -> (w144:dbl)
                          n101 = Compound Arithmetic op=MULTIPLY(w153, w138, 0.001 ("y")) -> (w135:dbl)
                          "Elaspsed Time [s]" <- w135
                          n102 = Build Array (concatenate)(w135, w148, w147, w146, w143, w144) -> (w150:dbl[])
                          n103 = call-poly <vilib>:"Write Delimited Spreadsheet.vi"("file path (dialog if empty)"=w152, "1D data"=w150, "append to file? (new file:F)"=TRUE, "delimiter (\\t)"="," ("delimiter (\\t)")) -> ()  [unwired: 10 in, 2 out]
                          n104 = Greater?(x=w135, y="Total Time") -> (0:w136:bool)
                          n105 = Multiply(x=w135, y=100.0) -> (x*y=w140:dbl)
                          n106 = Format Into String(format string="%06d", w140) -> (resulting string=w141:string)  [unwired: 2 in, 1 out]
                          n107 = shared-variable "PXI-Robot\\JointAngles.lvlib\\TimeStamp"(w141) -> ()  [unwired: 1 in, 1 out]
                          n108 = local read "Program Stop"() -> (w145:bool)
                          n109 = Not(x=w136) -> (.not. x?=w137:bool)
                          n110 = shared-variable "PXI-Robot\\JointAngles.lvlib\\Save Data"(w137) -> ()  [unwired: 1 in, 1 out]
                          n111 = Compound Arithmetic op=OR(w145, w136) -> (w155:bool)
                        }
                      }
                    }
                  }
                }
              }
            }
            n112 = local read "Program Stop"() -> (w87:bool)
          }
        }
        frame Enabled {
        }
      }
      n113 = timed-loop {
        timing: w72 -> [_]
        timing-out: [_] -> w71
        tunnel: w70 -> [w193]
        tunnel: w69 -> [w192]
        stop <- w188 stop-if-true
        # "2022-02-14 Kevin For Accurus"
        # "IOP Control Loop"
        n114 = node-c288() -> ()  [unwired: 1 in, 1 out]
        n115 = xnode "Read/Write Control"("FPGA VI Reference In"=w193, "error in"=w192) -> ("AI"=w187:i16[])  [unwired: 2 out]
        n116 = xnode "Read/Write Control"("FPGA VI Reference In"=w193, "error in"=w192, "Hydration On/Off (Connector2/DIO28)"="Hydration") -> ()  [unwired: 2 out]
        n117 = Array Subset(array=w187, index=0, length=4) -> (w184:i16[])
        n118 = Multiply(x=w184, y=0.00030517578125) -> (x*y=w182:dbl[])
        n119 = call "IOP Calibration.vi"("IOP Input [V]"=w182) -> ("IOP Output [mmHg]"=w172:dbl[])  [unwired: 10 in]
        "Pressure Reading" <- w172
        n120 = Index Array(array=w172, index=2) -> (element=w190:dbl)
        n121 = Array To Cluster(array=w172) -> (cluster=→"Pressure Plots":T17)
        n122 = shared-variable "PXI-Robot\\JointAngles.lvlib\\IOP Readings"(w172) -> ()  [unwired: 1 in, 1 out]
        n123 = local read "Max Limit [mmHg]"() -> (w189:dbl)
        n124 = global write "Global Variables.vi" "IOP Ctrl Engaged?"("PID ON/OFF") -> ()
        n125 = call "RisingEdge.vi"("Signal In"="PID ON/OFF") -> ("Rising Edge"=w179:bool)  [unwired: 10 in]
        n126 = case shown="False" "PID ON/OFF" {
          tunnel: "Target IOP" -> [_ w207]
          tunnel: w190 -> [_ w206]
          tunnel: w189 -> [w198 w201]
          tunnel: w179 -> [_ w205]
          tunnel: [w198 w201] -> w173
          tunnel: [w197 w200] -> w177
          frame False {
            n127 = In Range and Coerce(upper limit=w198, x="Vac Cmd [mmHg]", lower limit=0.0) -> (coerced(x)=w197:dbl)  [unwired: 1 out]
            n128 = To Single Precision Float(number=w197) -> (single precision float=w196:sgl)
            n129 = local write "Vac Cmd [mmHg]"(w196) -> ()
          }
          frame True {
            n130 = call "vacPIDantiWindup.vi"("Saturation U"=w201, "Saturation M"=w201, "Reset"=w205, "PID Gains"="IOP PID Gains", "Feedback"=w206, "Reference"=w207) -> ("Control"=w199:dbl)  [unwired: 5 in]
            n131 = To Single Precision Float(number=w199) -> (single precision float=w203:sgl)
            n132 = local write "Vac Cmd [mmHg]"(w203) -> ()
            n133 = In Range and Coerce(upper limit=w201, x=w199, lower limit=10.0) -> (coerced(x)=w200:dbl)  [unwired: 1 out]
          }
        }
        n134 = To Double Precision Float(number=w177) -> (double precision float=w174:dbl)
        n135 = Divide(x=w174, y=w173) -> (x/y=w171:dbl)
        n136 = Multiply(x=w171, y=78.0) -> (x*y=w169:dbl)
        n137 = local read "Program Stop"() -> (w188:bool)
        n138 = To Byte Integer(number=w169) -> (8bit integer=w178:i8)
        n139 = global write "Global Variables.vi" "vac digit cmd"(w178) -> ()
        n140 = node-c288() -> ()  [unwired: 1 in, 1 out]
      }
      n141 = while {
        tunnel: w80 -> [w319]
        tunnel: w83 -> [w318]
        tunnel: [w317] -> w74
        tunnel: [w316] -> w73
        shift-right: [w314] -> _
        shift-left: T11 {"Prev L1 to L4 Posit"=[0.0, 0.0, 0.0, 0.0], "Prev Stage Posit"=[100.0, 70.0, 30.0], "Prev OCT Z Posit"=0.0} ("Prev Posit Cluster") -> [w315]
        shift-right: [w312] -> _
        shift-left: 0 -> [w311]
        shift-right: [w310] -> _
        shift-left: T2 {"Traj Px Array"=[], "Traj Py Array"=[], "Traj Pz Array"=[], "Speed Array"=[], "Depth Array"=[]} ("Trajectory Cluster") -> [w308]
        shift-right: [w309] -> _
        shift-left: T4 {"X Grid"=[], "Y Grid"=[], "Za_true Surf"=[], "Iris Center"=[0.0, 5.0, 0.0], "Zp_true Surf"=[], "Pinv"=[[1.0, 0.0], [0.0, 1.0]], "za_true"=0.0, "za_work"=0.0, "zp_work"=0.0, "zp_true"=0.0} ("Eye Model Cluster") -> [w307]
        stop <- w313 stop-if-true
        # "State Execution Loop"
        n142 = Wait (ms)(milliseconds to wait=u32 10) -> ()  [unwired: 1 out]
        n143 = local read "Current System State"() -> (w306:T9)
        n144 = global read "Global Variables.vi" "armID"() -> (w305:i32)
        n145 = case shown="\"M/S Operation\"" w306 {
          tunnel: w319 -> [w321 w343 w358 w374 w391 w408 w448 w464 w478 w492]
          tunnel: w318 -> [w329 w342 w356 w371 w387 w404 w444 w460 w475 w489]
          tunnel: [w325 w338 w354 w373 w384 w420 w447 w459 w471 w488] -> w317
          tunnel: [w328 w340 w352 w367 w386 w422 w438 w456 w474 w486] -> w316
          tunnel: w315 -> [_ w337 w357 w369 w389 w405 w442 w462 w477 w491]
          tunnel: [w335 w339 w353 w368 w385 w421 w440 w458 w472 w487] -> w314
          tunnel: [0 ("Last Index") 0 ("Last Index") 0 ("Last Index") 0 ("Last Index") 0 ("Last Index") 0 w439 w457 w473 w500] -> w312
          tunnel: w311 -> [_ _ _ _ _ _ w443 w461 w476 w500]
          tunnel: [T2 {"Traj Px Array"=[], "Traj Py Array"=[], "Traj Pz Array"=[], "Speed Array"=[], "Depth Array"=[]} ("Trajectory Cluster") T2 {"Traj Px Array"=[], "Traj Py Array"=[], "Traj Pz Array"=[], "Speed Array"=[], "Depth Array"=[]} ("Trajectory Cluster") T2 {"Traj Px Array"=[], "Traj Py Array"=[], "Traj Pz Array"=[], "Speed Array"=[], "Depth Array"=[]} ("Trajectory Cluster") T2 {"Traj Px Array"=[], "Traj Py Array"=[], "Traj Pz Array"=[], "Speed Array"=[], "Depth Array"=[]} ("Trajectory Cluster") T2 {"Traj Px Array"=[], "Traj Py Array"=[], "Traj Pz Array"=[], "Speed Array"=[], "Depth Array"=[]} ("Trajectory Cluster") w419 w441 w454 w480 w499] -> w310
          tunnel: [T4 {"X Grid"=[], "Y Grid"=[], "Za_true Surf"=[], "Iris Center"=[0.0, 5.0, 0.0], "Zp_true Surf"=[], "Pinv"=[[1.0, 0.0], [0.0, 1.0]], "za_true"=0.0, "za_work"=0.0, "zp_work"=0.0, "zp_true"=0.0} ("Eye Model Cluster") T4 {"X Grid"=[], "Y Grid"=[], "Za_true Surf"=[], "Iris Center"=[0.0, 5.0, 0.0], "Zp_true Surf"=[], "Pinv"=[[1.0, 0.0], [0.0, 1.0]], "za_true"=0.0, "za_work"=0.0, "zp_work"=0.0, "zp_true"=0.0} ("Eye Model Cluster") T4 {"X Grid"=[], "Y Grid"=[], "Za_true Surf"=[], "Iris Center"=[0.0, 5.0, 0.0], "Zp_true Surf"=[], "Pinv"=[[1.0, 0.0], [0.0, 1.0]], "za_true"=0.0, "za_work"=0.0, "zp_work"=0.0, "zp_true"=0.0} ("Eye Model Cluster") T4 {"X Grid"=[], "Y Grid"=[], "Za_true Surf"=[], "Iris Center"=[0.0, 5.0, 0.0], "Zp_true Surf"=[], "Pinv"=[[1.0, 0.0], [0.0, 1.0]], "za_true"=0.0, "za_work"=0.0, "zp_work"=0.0, "zp_true"=0.0} ("Eye Model Cluster") T4 {"X Grid"=[], "Y Grid"=[], "Za_true Surf"=[], "Iris Center"=[0.0, 5.0, 0.0], "Zp_true Surf"=[], "Pinv"=[[1.0, 0.0], [0.0, 1.0]], "za_true"=0.0, "za_work"=0.0, "zp_work"=0.0, "zp_true"=0.0} ("Eye Model Cluster") w418 w445 w455 w470 w498] -> w309
          tunnel: w308 -> [_ _ _ _ _ _ w441 w454 w480 w499]
          tunnel: w307 -> [_ _ _ _ _ _ w445 w455 w470 w498]
          tunnel: w305 -> [w324 w336 w351 w366 w382 w398 w437 w453 w469 w485]
          frame "Homing", Default {
            n146 = call "Homing v2.vi"("Robot In"=w324, "error in"=w329, "ToolInsertionOffset"="Tool Offset [mm]", "ToolType"="Tool Type", "FPGA VI Reference In"=w321) -> ("error out"=w328:errorcluster, "Last Stage Posit"=w327:dbl[], "Last Joint Posit"=w326:dbl[], "FPGA VI Reference Out"=w325:refnum<k20>)  [unwired: 3 in]
            n147 = Bundle By Name(cluster=T11 {"Prev L1 to L4 Posit"=[-0.5409, 0.04404050915429177, -1.917656453185038, 0.02068014705882353], "Prev Stage Posit"=[6.001471972029684, 5.996134588585126, 6.000298217087839], "Prev OCT Z Posit"=-0.0} ("Prev Posit Cluster"), "Prev L1 to L4 Posit"=w326, "Prev Stage Posit"=w327, "Prev OCT Z Posit"=0.0) -> (w335:T11)
          }
          frame "M/S Initialization" {
            n148 = local read "Stage PID Cluster"() -> (w347:T5)
            n149 = local read "L1 to L4 PID Cluster"() -> (w346:T6)
            n150 = local read "OCT Z PID Gains"() -> (w345:cluster{"Kp":dbl, "Kd":dbl, "Ki":dbl})
            n151 = Bundle By Name(cluster=T15 {"L1 to L4 PID Cluster"={"L1 PID Gains"={"Kp"=0.005, "Kd"=0.5, "Ki"=0.0005}, "L2 PID Gains"={"Kp"=0.01, "Kd"=1.0, "Ki"=0.005}, "L3 PID Gains"={"Kp"=0.05, "Kd"=1.0, "Ki"=0.0005}, "L4 PID Gains"={"Kp"=0.1, "Kd"=0.1, "Ki"=0.0005}}, "Stage PID Cluster"={"Stage Z PID"={"Kp"=0.0005, "Kd"=0.001, "Ki"=0.0}, "Stage Y PID"={"Kp"=0.0003, "Kd"=0.01, "Ki"=0.0}, "Stage X PID"={"Kp"=0.0003, "Kd"=0.01, "Ki"=0.0}}, "OCT Z PID Gains"={"Kp"=0.0003, "Kd"=0.0001, "Ki"=0.01}} ("PID Cluster"), "Stage PID Cluster"=w347, "L1 to L4 PID Cluster"=w346, "OCT Z PID Gains"=w345) -> (w341:T15)
            n152 = call "MS Initialization v2.vi"("PID Cluster"=w341, "Robot In"=w336, "error in"=w342, "Prev Posit Cluster"=w337, "FPGA VI Reference In"=w343) -> ("error out"=w340:errorcluster, "Last Posit Cluster"=w339:T18, "FPGA VI Reference Out"=w338:refnum<k20>)  [unwired: 4 in]
          }
          frame "M/S Operation" {
            n153 = local read "Stage PID Cluster"() -> (w362:T5)
            n154 = local read "L1 to L4 PID Cluster"() -> (w361:T6)
            n155 = local read "OCT Z PID Gains"() -> (w360:cluster{"Kp":dbl, "Kd":dbl, "Ki":dbl})
            n156 = Bundle By Name(cluster=T15 {"L1 to L4 PID Cluster"={"L1 PID Gains"={"Kp"=0.005, "Kd"=0.5, "Ki"=0.0005}, "L2 PID Gains"={"Kp"=0.01, "Kd"=1.0, "Ki"=0.005}, "L3 PID Gains"={"Kp"=0.05, "Kd"=1.0, "Ki"=0.0005}, "L4 PID Gains"={"Kp"=0.1, "Kd"=0.1, "Ki"=0.0005}}, "Stage PID Cluster"={"Stage Z PID"={"Kp"=0.0005, "Kd"=0.001, "Ki"=0.0}, "Stage Y PID"={"Kp"=0.0003, "Kd"=0.01, "Ki"=0.0}, "Stage X PID"={"Kp"=0.0003, "Kd"=0.01, "Ki"=0.0}}, "OCT Z PID Gains"={"Kp"=0.0003, "Kd"=0.0001, "Ki"=0.01}} ("PID Cluster"), "Stage PID Cluster"=w362, "L1 to L4 PID Cluster"=w361, "OCT Z PID Gains"=w360) -> (w355:T15)
            n157 = call "MS Operation v2.vi"("PID Cluster"=w355, "Robot In"=w351, "error in"=w356, "Prev Posit Cluster"=w357, "FPGA VI Reference In"=w358) -> ("error out"=w352:errorcluster, "Last Posit Cluster"=w353:T18, "FPGA VI Reference Out"=w354:refnum<k20>)  [unwired: 4 in]
          }
          frame "Aiming" {
            n158 = local read "Aiming Pt"() -> (w370:dbl[])
            n159 = local read "Stage PID Cluster"() -> (w378:T5)
            n160 = local read "L1 to L4 PID Cluster"() -> (w377:T6)
            n161 = local read "OCT Z PID Gains"() -> (w375:cluster{"Kp":dbl, "Kd":dbl, "Ki":dbl})
            n162 = Bundle By Name(cluster=T15 {"L1 to L4 PID Cluster"={"L1 PID Gains"={"Kp"=0.005, "Kd"=0.5, "Ki"=0.0005}, "L2 PID Gains"={"Kp"=0.01, "Kd"=1.0, "Ki"=0.005}, "L3 PID Gains"={"Kp"=0.05, "Kd"=1.0, "Ki"=0.0005}, "L4 PID Gains"={"Kp"=0.1, "Kd"=0.1, "Ki"=0.0005}}, "Stage PID Cluster"={"Stage Z PID"={"Kp"=0.0005, "Kd"=0.001, "Ki"=0.0}, "Stage Y PID"={"Kp"=0.0003, "Kd"=0.01, "Ki"=0.0}, "Stage X PID"={"Kp"=0.0003, "Kd"=0.01, "Ki"=0.0}}, "OCT Z PID Gains"={"Kp"=0.0003, "Kd"=0.0001, "Ki"=0.01}} ("PID Cluster"), "Stage PID Cluster"=w378, "L1 to L4 PID Cluster"=w377, "OCT Z PID Gains"=w375) -> (w372:T15)
            n163 = call "Aiming v2.vi"("PID Cluster"=w372, "Robot In"=w366, "error in"=w371, "Aiming Pt"=w370, "Prev Posit Cluster"=w369, "FPGA VI Reference In"=w374) -> ("error out"=w367:errorcluster, "Last Posit Cluster"=w368:T18, "FPGA VI Reference Out"=w373:refnum<k20>)  [unwired: 3 in]
          }
          frame "Engaging" {
            n164 = local read "Engage Pt"() -> (w388:dbl[])
            n165 = local read "Stage PID Cluster"() -> (w394:T5)
            n166 = local read "L1 to L4 PID Cluster"() -> (w393:T6)
            n167 = local read "OCT Z PID Gains"() -> (w392:cluster{"Kp":dbl, "Kd":dbl, "Ki":dbl})
            n168 = Bundle By Name(cluster=T15 {"L1 to L4 PID Cluster"={"L1 PID Gains"={"Kp"=0.005, "Kd"=0.5, "Ki"=0.0005}, "L2 PID Gains"={"Kp"=0.01, "Kd"=1.0, "Ki"=0.005}, "L3 PID Gains"={"Kp"=0.05, "Kd"=1.0, "Ki"=0.0005}, "L4 PID Gains"={"Kp"=0.1, "Kd"=0.1, "Ki"=0.0005}}, "Stage PID Cluster"={"Stage Z PID"={"Kp"=0.0005, "Kd"=0.001, "Ki"=0.0}, "Stage Y PID"={"Kp"=0.0003, "Kd"=0.01, "Ki"=0.0}, "Stage X PID"={"Kp"=0.0003, "Kd"=0.01, "Ki"=0.0}}, "OCT Z PID Gains"={"Kp"=0.0003, "Kd"=0.0001, "Ki"=0.01}} ("PID Cluster"), "Stage PID Cluster"=w394, "L1 to L4 PID Cluster"=w393, "OCT Z PID Gains"=w392) -> (w390:T15)
            n169 = call "Engaging v2.vi"("PID Cluster"=w390, "Robot In"=w382, "error in"=w387, "Engage Pt"=w388, "Prev Posit Cluster"=w389, "FPGA VI Reference In"=w391) -> ("error out"=w386:errorcluster, "Last Posit Cluster"=w385:T18, "FPGA VI Reference Out"=w384:refnum<k20>)  [unwired: 3 in]
          }
          frame "Trajectory Loading" {
            n170 = local read "Stage PID Cluster"() -> (w412:T5)
            n171 = local read "L1 to L4 PID Cluster"() -> (w411:T6)
            n172 = local read "OCT Z PID Gains"() -> (w410:cluster{"Kp":dbl, "Kd":dbl, "Ki":dbl})
            n173 = Bundle By Name(cluster=T15 {"L1 to L4 PID Cluster"={"L1 PID Gains"={"Kp"=0.005, "Kd"=0.5, "Ki"=0.0005}, "L2 PID Gains"={"Kp"=0.01, "Kd"=1.0, "Ki"=0.005}, "L3 PID Gains"={"Kp"=0.05, "Kd"=1.0, "Ki"=0.0005}, "L4 PID Gains"={"Kp"=0.1, "Kd"=0.1, "Ki"=0.0005}}, "Stage PID Cluster"={"Stage Z PID"={"Kp"=0.0005, "Kd"=0.001, "Ki"=0.0}, "Stage Y PID"={"Kp"=0.0003, "Kd"=0.01, "Ki"=0.0}, "Stage X PID"={"Kp"=0.0003, "Kd"=0.01, "Ki"=0.0}}, "OCT Z PID Gains"={"Kp"=0.0003, "Kd"=0.0001, "Ki"=0.01}} ("PID Cluster"), "Stage PID Cluster"=w412, "L1 to L4 PID Cluster"=w411, "OCT Z PID Gains"=w410) -> (w407:T15)
            n174 = call "Trajectory Loading v2.vi"("PID Cluster"=w407, "Robot In"=w398, "error in"=w404, "Prev Posit Cluster"=w405, "FPGA VI Reference In"=w408) -> ("Eye Model Cluster"=w400:T4, "Trajectory Cluster"=w401:T2, "Last Posit Cluster"=w402:T18, "FPGA VI Reference Out"=w403:refnum<k20>, "error out"=w406:errorcluster, "First Trk Pt"=→"First Trk Pt":dbl[])  [unwired: 1 in]
            n175 = flat-sequence {
              tunnel: w401 -> [w429]
              tunnel: w400 -> [w430]
              tunnel: w406 -> [w428]
              tunnel: [w428] -> w417
              tunnel: w402 -> [w427]
              tunnel: [w427] -> w416
              tunnel: w403 -> [w426]
              tunnel: [w426] -> w415
              tunnel: [w425] -> w414
              tunnel: w401 -> [w425]
              tunnel: w400 -> [w424]
              tunnel: [w424] -> w413
              tunnel: [w435] -> w422
              tunnel: w417 -> [w435]
              tunnel: [w434] -> w421
              tunnel: w416 -> [w434]
              tunnel: w415 -> [w433]
              tunnel: [w433] -> w420
              tunnel: w414 -> [w432]
              tunnel: w413 -> [w431]
              tunnel: [w432] -> w419
              tunnel: [w431] -> w418
              frame #0 {
                "Eye Model Cluster" <- w430
                "Trajectory Cluster" <- w429
              }
              frame #1 {
                "Update Mdl & Traj" <- TRUE
              }
            }
          }
          frame "Tracking Initialization" {
            n176 = local read "Stage PID Cluster"() -> (w452:T5)
            n177 = local read "L1 to L4 PID Cluster"() -> (w451:T6)
            n178 = local read "OCT Z PID Gains"() -> (w449:cluster{"Kp":dbl, "Kd":dbl, "Ki":dbl})
            n179 = Bundle By Name(cluster=T15 {"L1 to L4 PID Cluster"={"L1 PID Gains"={"Kp"=0.005, "Kd"=0.5, "Ki"=0.0005}, "L2 PID Gains"={"Kp"=0.01, "Kd"=1.0, "Ki"=0.005}, "L3 PID Gains"={"Kp"=0.05, "Kd"=1.0, "Ki"=0.0005}, "L4 PID Gains"={"Kp"=0.1, "Kd"=0.1, "Ki"=0.0005}}, "Stage PID Cluster"={"Stage Z PID"={"Kp"=0.0005, "Kd"=0.001, "Ki"=0.0}, "Stage Y PID"={"Kp"=0.0003, "Kd"=0.01, "Ki"=0.0}, "Stage X PID"={"Kp"=0.0003, "Kd"=0.01, "Ki"=0.0}}, "OCT Z PID Gains"={"Kp"=0.0003, "Kd"=0.0001, "Ki"=0.01}} ("PID Cluster"), "Stage PID Cluster"=w452, "L1 to L4 PID Cluster"=w451, "OCT Z PID Gains"=w449) -> (w446:T15)
            n180 = call "Tracking Initialization v2.vi"("Eye Model Cluster"=w445, "Trajectory Cluster"=w441, "PID Cluster"=w446, "Robot In"=w437, "error in"=w444, "Prev Index"=w443, "Prev Posit Cluster"=w442, "FPGA VI Reference In"=w448) -> ("error out"=w438:errorcluster, "Last Index"=w439:i32, "Last Posit Cluster"=w440:T18, "FPGA VI Reference Out"=w447:refnum<k20>)
          }
          frame "Tracking" {
            n181 = local read "Stage PID Cluster"() -> (w468:T5)
            n182 = local read "L1 to L4 PID Cluster"() -> (w467:T6)
            n183 = local read "OCT Z PID Gains"() -> (w466:cluster{"Kp":dbl, "Kd":dbl, "Ki":dbl})
            n184 = Bundle By Name(cluster=T15 {"L1 to L4 PID Cluster"={"L1 PID Gains"={"Kp"=0.005, "Kd"=0.5, "Ki"=0.0005}, "L2 PID Gains"={"Kp"=0.01, "Kd"=1.0, "Ki"=0.005}, "L3 PID Gains"={"Kp"=0.05, "Kd"=1.0, "Ki"=0.0005}, "L4 PID Gains"={"Kp"=0.1, "Kd"=0.1, "Ki"=0.0005}}, "Stage PID Cluster"={"Stage Z PID"={"Kp"=0.0005, "Kd"=0.001, "Ki"=0.0}, "Stage Y PID"={"Kp"=0.0003, "Kd"=0.01, "Ki"=0.0}, "Stage X PID"={"Kp"=0.0003, "Kd"=0.01, "Ki"=0.0}}, "OCT Z PID Gains"={"Kp"=0.0003, "Kd"=0.0001, "Ki"=0.01}} ("PID Cluster"), "Stage PID Cluster"=w468, "L1 to L4 PID Cluster"=w467, "OCT Z PID Gains"=w466) -> (w463:T15)
            n185 = call "Tracking v2.vi"("Robot In"=w453, "Trajectory Cluster"=w454, "PID Cluster"=w463, "Eye Model Cluster"=w455, "error in"=w460, "Resume Index"=w461, "Prev Posit Cluster"=w462, "FPGA VI Reference In"=w464) -> ("error out"=w456:errorcluster, "Leave Index"=w457:i32, "Last Posit Cluster"=w458:T18, "FPGA VI Reference Out"=w459:refnum<k20>)
          }
          frame "Rerouting" {
            n186 = local read "Stage PID Cluster"() -> (w483:T5)
            n187 = local read "L1 to L4 PID Cluster"() -> (w482:T6)
            n188 = local read "OCT Z PID Gains"() -> (w481:cluster{"Kp":dbl, "Kd":dbl, "Ki":dbl})
            n189 = Bundle By Name(cluster=T15 {"L1 to L4 PID Cluster"={"L1 PID Gains"={"Kp"=0.005, "Kd"=0.5, "Ki"=0.0005}, "L2 PID Gains"={"Kp"=0.01, "Kd"=1.0, "Ki"=0.005}, "L3 PID Gains"={"Kp"=0.05, "Kd"=1.0, "Ki"=0.0005}, "L4 PID Gains"={"Kp"=0.1, "Kd"=0.1, "Ki"=0.0005}}, "Stage PID Cluster"={"Stage Z PID"={"Kp"=0.0005, "Kd"=0.001, "Ki"=0.0}, "Stage Y PID"={"Kp"=0.0003, "Kd"=0.01, "Ki"=0.0}, "Stage X PID"={"Kp"=0.0003, "Kd"=0.01, "Ki"=0.0}}, "OCT Z PID Gains"={"Kp"=0.0003, "Kd"=0.0001, "Ki"=0.01}} ("PID Cluster"), "Stage PID Cluster"=w483, "L1 to L4 PID Cluster"=w482, "OCT Z PID Gains"=w481) -> (w479:T15)
            n190 = call "Rerouting v2.vi"("Eye Model Cluster"=w470, "Trajectory Cluster"=w480, "PID Cluster"=w479, "Robot In"=w469, "error in"=w475, "Prev Index"=w476, "Prev Posit Cluster"=w477, "FPGA VI Reference In"=w478) -> ("error out"=w474:errorcluster, "Last Index"=w473:i32, "Last Posit Cluster"=w472:T18, "FPGA VI Reference Out"=w471:refnum<k20>)
          }
          frame "Regulation" {
            n191 = local read "Engage Pt"() -> (w490:dbl[])
            n192 = local read "Stage PID Cluster"() -> (w496:T5)
            n193 = local read "L1 to L4 PID Cluster"() -> (w495:T6)
            n194 = local read "OCT Z PID Gains"() -> (w494:cluster{"Kp":dbl, "Kd":dbl, "Ki":dbl})
            n195 = Bundle By Name(cluster=T15 {"L1 to L4 PID Cluster"={"L1 PID Gains"={"Kp"=0.005, "Kd"=0.5, "Ki"=0.0005}, "L2 PID Gains"={"Kp"=0.01, "Kd"=1.0, "Ki"=0.005}, "L3 PID Gains"={"Kp"=0.05, "Kd"=1.0, "Ki"=0.0005}, "L4 PID Gains"={"Kp"=0.1, "Kd"=0.1, "Ki"=0.0005}}, "Stage PID Cluster"={"Stage Z PID"={"Kp"=0.0005, "Kd"=0.001, "Ki"=0.0}, "Stage Y PID"={"Kp"=0.0003, "Kd"=0.01, "Ki"=0.0}, "Stage X PID"={"Kp"=0.0003, "Kd"=0.01, "Ki"=0.0}}, "OCT Z PID Gains"={"Kp"=0.0003, "Kd"=0.0001, "Ki"=0.01}} ("PID Cluster"), "Stage PID Cluster"=w496, "L1 to L4 PID Cluster"=w495, "OCT Z PID Gains"=w494) -> (w493:T15)
            n196 = call "Regulation v2.vi"("PID Cluster"=w493, "Robot In"=w485, "error in"=w489, "Engage Pt"=w490, "Prev Posit Cluster"=w491, "FPGA VI Reference In"=w492) -> ("error out"=w486:errorcluster, "Last Posit Cluster"=w487:T18, "FPGA VI Reference Out"=w488:refnum<k20>)  [unwired: 3 in]
          }
        }
        n197 = local read "Program Stop"() -> (w313:bool)
      }
      n198 = while {
        shift-right: [w213] -> _
        shift-left: errorcluster {"status"=FALSE, "code"=0, "source"=""} ("error IO") -> [w218]
        stop <- w216 stop-if-true
        # "Eye Model and Trajectory Generation"
        n199 = Wait (ms)(milliseconds to wait=u32 100) -> ()  [unwired: 1 out]
        n200 = event shown="[3] \"Gen Traj\": Mouse Up" {
          selector: _ -> [_ _ _ _]
          dyn-events: _ -> [_ _ _ _]
          timeout: 100 -> [_ _ _ _]
          tunnel: [w224 w225 errorcluster {"status"=FALSE, "code"=0, "source"=""} ("error IO") w259] -> w213
          tunnel: w218 -> [w224 w228 _ w259]
          tunnel: "SCAN_NO" -> [_ w229 _ w258]
          event Timeout {
            # "timeout"
            n201 = event-data() -> ()  [unwired: 1 in, 1 out]
          }
          event "Process VSCAN": Value Change {
            # "run ML script to segment the vscan (ACh or PC)"
            n202 = event-data() -> ()  [unwired: 1 in, 2 out]
            n203 = flat-sequence {
              tunnel: w229 -> [w233]
              tunnel: w228 -> [w232]
              tunnel: [w231] -> w227
              tunnel: w227 -> [w237]
              tunnel: [w237] -> w226
              tunnel: w226 -> [w240]
              tunnel: [w239] -> w225
              frame #0 {
                n204 = disable-structure shown="Disabled" {
                  disable-tunnel: w233 -> [w236 _]
                  disable-tunnel: w232 -> [w235 _]
                  disable-tunnel: [w234 _] -> w231
                  frame Disabled {
                    n205 = script code="% 2021-09-20 MJG \n% Segment vscan, generate {OCT} [mm] plot, and save all model parameters\ncd('D:\\IRISSoft LV2016 beta\\Host Demo\\Traj\\BuildModel\\matlab');\n\nclear processVSCAN_v3;\nprocessVSCAN_v3(SCAN_NO_ACh);"("??"=w235, "SCAN_NO_ACh"=w236) -> ("??"=w234:errorcluster)
                  }
                  frame Enabled {
                  }
                }
              }
              frame #1 {
                n206 = disable-structure shown="Disabled" {
                  frame Disabled {
                    w238 = dbl[] [0.0, 0.0, 0.0, 0.0] ("First Trk Pt 2")
                    n207 = global write "Global Variables.vi" "xPC"(w238) -> ()
                    n208 = global write "Global Variables.vi" "yPC"(w238) -> ()
                    n209 = global write "Global Variables.vi" "zPC"(w238) -> ()
                    n210 = global write "Global Variables.vi" "xACh"(w238) -> ()
                    n211 = global write "Global Variables.vi" "yACh"(w238) -> ()
                    n212 = global write "Global Variables.vi" "zACh"(w238) -> ()
                  }
                  frame Enabled {
                  }
                }
              }
              frame #2 {
                n213 = disable-structure shown="Disabled" {
                  disable-tunnel: w240 -> [w245 _]
                  disable-tunnel: [w244 _] -> w239
                  frame Disabled {
                    n214 = local read "SCAN_NO"() -> (w249:string)
                    n215 = script code="cd('D:\\IRISSoft LV2016 beta\\Host Demo\\Traj');\nclear visMdlInLV;\n[xACh, yACh, zACh, xIris, yIris, zIris, xPC, yPC, zPC] = visMdlInLV(SCAN_NO);"("??"=w245, "SCAN_NO"=w249) -> ("??"=w244:errorcluster, "xACh"=w250:dbl[], "yACh"=w251:dbl[], "zACh"=w252:dbl[], "xPC"=w248:dbl[], "yPC"=w247:dbl[], "zPC"=w246:dbl[], "xIris"=w243:dbl[], "yIris"=w242:dbl[], "zIris"=w241:dbl[])
                    n216 = global write "Global Variables.vi" "xACh"(w250) -> ()
                    n217 = global write "Global Variables.vi" "yACh"(w251) -> ()
                    n218 = global write "Global Variables.vi" "zACh"(w252) -> ()
                    n219 = global write "Global Variables.vi" "xIris"(w243) -> ()
                    n220 = global write "Global Variables.vi" "yIris"(w242) -> ()
                    n221 = global write "Global Variables.vi" "zIris"(w241) -> ()
                    n222 = global write "Global Variables.vi" "xPC"(w248) -> ()
                    n223 = global write "Global Variables.vi" "yPC"(w247) -> ()
                    n224 = global write "Global Variables.vi" "zPC"(w246) -> ()
                  }
                  frame Enabled {
                  }
                }
              }
            }
            n225 = disable-structure shown="Disabled" {
              frame Disabled {
                "Model Created" <- TRUE ("Model Created")
              }
              frame Enabled {
              }
            }
          }
          event "Restart": Mouse Up {
            n226 = event-data() -> ()  [unwired: 1 in, 2 out]
            n227 = disable-structure shown="Disabled" {
              frame Disabled {
                n228 = local write "Model Created"(FALSE ("Model Created")) -> ()
              }
              frame Enabled {
              }
            }
          }
          event "Gen Traj": Mouse Up {
            # "Generate trajectory"
            n229 = event-data() -> ()  [unwired: 1 in, 2 out]
            n230 = flat-sequence {
              tunnel: w258 -> [w261]
              tunnel: [w261] -> w257
              tunnel: w257 -> [w262]
              tunnel: [w262] -> w256
              tunnel: w256 -> [w270]
              tunnel: [w270] -> w255
              tunnel: w255 -> [w295]
              frame #0 {
                w260 = dbl[] [0.0, 0.0, 0.0, 0.0] ("First Trk Pt 2")
                n231 = global write "Global Variables.vi" "xTraj"(w260) -> ()
                n232 = global write "Global Variables.vi" "yTraj"(w260) -> ()
                n233 = global write "Global Variables.vi" "zTraj"(w260) -> ()
                n234 = global write "Global Variables.vi" "xPC"(w260) -> ()
                n235 = global write "Global Variables.vi" "yPC"(w260) -> ()
                n236 = global write "Global Variables.vi" "zPC"(w260) -> ()
                n237 = global write "Global Variables.vi" "xIris"(w260) -> ()
                n238 = global write "Global Variables.vi" "yIris"(w260) -> ()
                n239 = global write "Global Variables.vi" "zIris"(w260) -> ()
                n240 = global write "Global Variables.vi" "xACh"(w260) -> ()
                n241 = global write "Global Variables.vi" "yACh"(w260) -> ()
                n242 = global write "Global Variables.vi" "zACh"(w260) -> ()
              }
              frame #1 {
                n243 = call "Host Gen Trajectory.vi"("Trajectory Pattern"="Pattern", "Depth Ctrl Array\n(% Thickness)"="Depth Ctrl Array\n(% Thickness)", "Traj Scale Radius from Pupil Radius (Between 0 and 1)"="Radial Scale", "Traj Offset from Pupil Center [mm]"="Offset", "SCAN_NO"=w262) -> ("zVisTraj"=w268:dbl[], "yVisTraj"=w267:dbl[], "xVisTraj"=w269:dbl[])  [unwired: 4 in]
                n244 = global write "Global Variables.vi" "xTraj"(w269) -> ()
                n245 = global write "Global Variables.vi" "yTraj"(w267) -> ()
                n246 = global write "Global Variables.vi" "zTraj"(w268) -> ()
              }
              frame #2 {
                w273 = 0  # Counter
                n247 = shared-variable "PXI-Robot\\JointAngles.lvlib\\Traj Px Array"() -> (w276:dbl[])  [unwired: 1 in, 1 out]
                n248 = shared-variable "PXI-Robot\\JointAngles.lvlib\\Traj Py Array"() -> (w275:dbl[])  [unwired: 1 in, 1 out]
                n249 = shared-variable "PXI-Robot\\JointAngles.lvlib\\Traj Pz Array"() -> (w274:dbl[])  [unwired: 1 in, 1 out]
                n250 = global read "Global Variables.vi" "armID"() -> (w278:i32)
                n251 = Array Size(array=w276) -> (size(s)=w277:i32)
                n252 = for {
                  N: w277 -> [_]
                  tunnel: w278 -> [w291]
                  tunnel: w276 -> [w290] mode=indexing
                  tunnel: w275 -> [w289] mode=indexing
                  tunnel: w274 -> [w288] mode=indexing
                  shift-right: [w279] -> w272
                  shift-left: w273 -> [w280]
                  n253 = call "Inverse Kinematics.vi"("isToolTipInsideEye"=TRUE, "armID"=w291, "z"=w288, "y"=w289, "x"=w290) -> ("j3"=w283:dbl, "j2"=w284:dbl, "j1"=w285:dbl)  [unwired: 3 in, 1 out]
                  n254 = Build Array(w285, w284, w283) -> (w282:dbl[])
                  n255 = global read "Global Variables.vi" "joint limits"() -> (w286:dbl[][])
                  n256 = call "Joint Saturation Demo.vi"("Joint Bounds [Deg/mm]"=w286, "Ref Array [Deg/mm]"=w282) -> ("Out of Bound?"=w281:bool)  [unwired: 8 in, 1 out]
                  n257 = case shown="True" w281 {
                    tunnel: w280 -> [w292 w294]
                    tunnel: [w292 w293] -> w279
                    frame False {
                    }
                    frame True {
                      n258 = Increment(x=w294) -> (x+1=w293:i32)
                    }
                  }
                }
                n259 = Not Equal To 0?(x=w272) -> (x != 0?=→"Trajectory OOB":bool)
              }
              frame #3 {
                n260 = script code="cd('D:\\IRISSoft LV2016 beta\\Host Demo\\Traj');\nclear visMdlInLV;\n[xACh, yACh, zACh, xIris, yIris, zIris, xPC, yPC, zPC] = visMdlInLV(SCAN_NO);"("SCAN_NO"=w295) -> ("xACh"=w302:dbl[], "yACh"=w303:dbl[], "zACh"=w304:dbl[], "xPC"=w301:dbl[], "yPC"=w300:dbl[], "zPC"=w299:dbl[], "xIris"=w298:dbl[], "yIris"=w297:dbl[], "zIris"=w296:dbl[])  [unwired: 1 in, 1 out]
                n261 = global write "Global Variables.vi" "xACh"(w302) -> ()
                n262 = global write "Global Variables.vi" "yACh"(w303) -> ()
                n263 = global write "Global Variables.vi" "zACh"(w304) -> ()
                n264 = global write "Global Variables.vi" "xIris"(w298) -> ()
                n265 = global write "Global Variables.vi" "yIris"(w297) -> ()
                n266 = global write "Global Variables.vi" "zIris"(w296) -> ()
                n267 = global write "Global Variables.vi" "xPC"(w301) -> ()
                n268 = global write "Global Variables.vi" "yPC"(w300) -> ()
                n269 = global write "Global Variables.vi" "zPC"(w299) -> ()
              }
            }
          }
        }
        "Generation Error" <- w213
        n270 = case shown="True" "Use Online Scan" {
          frame False {
            # "User specified SCAN_NO"
          }
          frame True {
            # "Use the SCAN_NO from OCT computer"
            n271 = shared-variable "PXI-Robot\\JointAngles.lvlib\\SCAN_NO"() -> (w223:string)  [unwired: 1 in, 1 out]
            n272 = local write "SCAN_NO"(w223) -> ()
          }
        }
        n273 = shared-variable "PXI-Robot\\JointAngles.lvlib\\Scan Done"() -> (w214:bool)  [unwired: 1 in, 1 out]
        n274 = case shown="True" w214 {
          frame False {
          }
          frame True {
            n275 = property on="Process VSCAN" class="Bool (strict)"() -> ("Value"=w222:bool)  [unwired: 2 in, 2 out]
            n276 = Not(x=w222) -> (.not. x?=w221:bool)
            n277 = property on="Process VSCAN" class="Bool (strict)"("Val(Sgnl)"=w221) -> ()  [unwired: 2 in, 2 out]
            n278 = shared-variable "PXI-Robot\\JointAngles.lvlib\\Scan Done"(FALSE ("Scan Done")) -> ()  [unwired: 1 in, 1 out]
          }
        }
        n279 = local read "Program Stop"() -> (w216:bool)
      }
      n280 = while {
        tunnel: w85 -> [w532]
        tunnel: [w531] -> w84
        stop <- w542 stop-if-true
        # "2022-02-15 Kevin:\nIRISS V2 XYZ stage jnts are flipped"
        # "Indicator Loop"
        n281 = Wait (ms)(milliseconds to wait=u32 100) -> ()  [unwired: 1 out]
        n282 = global read "Global Variables.vi" "armID"() -> (w507:i32)
        n283 = global read "Global Variables.vi" "L1 to L4 cmd Posit"() -> (w512:dbl[])
        n284 = call "IRISS V2 Get Joint Out.vi"("Left or Right Arm"=w507) -> ("grasp"=→"Grasp out":dbl, "Joint Out Posit"=w506:dbl[])  [unwired: 3 in]
        "Joint Out" <- w506
        n285 = call "IRISS V2 Get XYZ Out.vi"("Left or Right Arm"=w507) -> ("XYZ Out Posit"=w505:dbl[])  [unwired: 3 in, 1 out]
        "Tip out Posit" <- w505
        n286 = Index Array(array=w512, index #1=0 ("index"), index #2=1 ("index"), index #3=2 ("index"), index #4=3 ("index")) -> (element #1=w509:dbl, element #2=w510:dbl, element #3=w508:dbl)  [unwired: 1 out]
        n287 = call "Forward Kinematics.vi"("j3"=w508, "j2"=w510, "j1"=w509, "armID"=w507) -> ("XYZ Out Array"=→"Tip cmd Posit":dbl[])  [unwired: 7 in]
        n288 = shared-variable "PXI-Robot\\JointAngles.lvlib\\L1 to L4 Out"(w506) -> ()  [unwired: 1 in, 1 out]
        n289 = shared-variable "PXI-Robot\\JointAngles.lvlib\\ToolTipPosition"(w505) -> ()  [unwired: 1 in, 1 out]
        n290 = global read "Global Variables.vi" "Stage cmd Posit"() -> (w541:dbl[])
        n291 = global read "Global Variables.vi" "Stage out Posit"() -> (w503:dbl[])
        n292 = global read "Global Variables.vi" "OCT Z out Posit"() -> (→"OCT Z out [mm]":dbl)
        n293 = Reverse 1D Array(array=w503) -> (reversed array=w502:dbl[])
        "XYZ Stage Out" <- w502
        n294 = Index Array(array=w541, index #1=0 ("index"), index #2=1 ("index"), index #3=2 ("index")) -> (element #1=→"X Stage cmd [mm]":dbl, element #2=→"Y Stage cmd [mm]":dbl, element #3=→"Z Stage cmd [mm]":dbl)  [unwired: 1 in, 1 out]
        n295 = Index Array(array=w502) -> (element #3=w501:dbl)  [unwired: 3 in, 2 out]
        n296 = shared-variable "PXI-Robot\\JointAngles.lvlib\\Stage Z Out"(w501) -> ()  [unwired: 1 in, 1 out]
        n297 = global read "Global Variables.vi" "irrigate"() -> (→"Irrigation Engaged?":bool)
        n298 = global read "Global Variables.vi" "vac digit cmd"() -> (w521:i8)
        n299 = global read "Global Variables.vi" "max limit [mmHg]"() -> (w518:dbl)
        n300 = global read "Global Variables.vi" "Robot Status Array"() -> (→"Robot Status Array":bool[])
        n301 = global read "Global Variables.vi" "Robot Home Status"() -> (→"Status 2":bool[])
        n302 = global read "Global Variables.vi" "Receive Count"() -> (→"Receive Count":u64)
        n303 = global read "Global Variables.vi" "Send Count"() -> (→"Send Count":u64)
        n304 = Divide(x=w521, y=i8 78) -> (x/y=w519:dbl)
        n305 = Multiply(x=w519, y=w518) -> (x*y=→"Value [mmHg]" →"Vacuum Force [mmHg]  2":dbl)
        n306 = global write "var_OCTzHomeDir.vi" "OCTz Home Dir"("OCTz Home Dir") -> ()
        n307 = shared-variable "PXI-Robot\\JointAngles.lvlib\\RemoteSenderEngaged"() -> (→"Remote sender engaged":bool)  [unwired: 1 in, 1 out]
        n308 = shared-variable "PXI-Robot\\JointAngles.lvlib\\EmergencyAlarmBit"() -> (→"Emergency alarm":bool)  [unwired: 1 in, 1 out]
        n309 = global read "Global Variables.vi" "assign pt out of bound"() -> (→"Asgn Pt Out of Bound":bool)
        n310 = global read "Global Variables.vi" "current run no."() -> (→"Current Run No.":u8)
        n311 = global read "Global Variables.vi" "tracking timer"() -> (w534:i32)
        n312 = global read "Global Variables.vi" "state changing"() -> (→"State changing":bool)
        n313 = global read "Global Variables.vi" "state flag array"() -> (→"State Flag Array":bool[])
        n314 = Divide(x=w534, y=10) -> (x/y=→"Timer":dbl)
        n315 = flat-sequence {
          frame #0 {
            w570 = sgl[] [0.0, 0.0]  # RCMy
            w569 = sgl[] [0.0, 0.0]  # RCMz
            w571 = sgl[] [0.0, 0.0]  # RCMx
            # "3D Visualization"
            n316 = disable-structure shown="Disabled" {
              disable-tunnel: [w580 _] -> w559
              frame Disabled {
                n317 = global read "Global Variables.vi" "xPC"() -> (w578:dbl[])
                n318 = global read "Global Variables.vi" "yPC"() -> (w577:dbl[])
                n319 = global read "Global Variables.vi" "zPC"() -> (w576:dbl[])
                n320 = call-poly <vilib>:"Plot Helper.vi"("Plot ID"=2, "z vector"=w576, "y vector"=w577, "x vector"=w578) -> ("3D Plot lvclass Array out"=w585:refnum<class "3D Plot Datatype.lvclass">[])  [unwired: 2 in, 5 out]
                n321 = global read "Global Variables.vi" "xACh"() -> (w583:dbl[])
                n322 = global read "Global Variables.vi" "yACh"() -> (w582:dbl[])
                n323 = global read "Global Variables.vi" "zACh"() -> (w581:dbl[])
                n324 = call-poly <vilib>:"Plot Helper.vi"("Plot ID"=3, "z vector"=w581, "y vector"=w582, "x vector"=w583, "3D Plot lvclass Array in"=w585) -> ("3D Plot lvclass Array out"=w580:refnum<class "3D Plot Datatype.lvclass">[])  [unwired: 1 in, 5 out]
              }
              frame Enabled {
              }
            }
            n325 = local read "Tip out Posit"() -> (w563:dbl[])
            n326 = call "Vis Interpolate Points.vi"("Tip out Posit"=w563) -> ("Z"=w560:dbl[], "Y"=w561:dbl[], "X"=w562:dbl[])  [unwired: 4 in]
            n327 = call-poly <vilib>:"Plot Helper.vi"("Plot ID"=1, "z vector"=w560, "y vector"=w561, "x vector"=w562, "3D Plot lvclass Array in"=w559) -> ("3D Plot lvclass Array out"=w553:refnum<class "3D Plot Datatype.lvclass">[])  [unwired: 1 in, 5 out]
            n328 = global read "Global Variables.vi" "xTraj"() -> (w554:dbl[])
            n329 = global read "Global Variables.vi" "yTraj"() -> (w555:dbl[])
            n330 = global read "Global Variables.vi" "zTraj"() -> (w556:dbl[])
            n331 = call-poly <vilib>:"Plot Helper.vi"("Plot ID"=4, "z vector"=w556, "y vector"=w555, "x vector"=w554, "3D Plot lvclass Array in"=w553) -> ("3D Plot lvclass Array out"=w551:refnum<class "3D Plot Datatype.lvclass">[])  [unwired: 1 in, 5 out]
            n332 = disable-structure shown="Enabled" {
              disable-tunnel: w551 -> [w587 w592]
              disable-tunnel: [w586 w592] -> w550
              frame Disabled {
                n333 = global read "Global Variables.vi" "xIris"() -> (w591:dbl[])
                n334 = global read "Global Variables.vi" "yIris"() -> (w590:dbl[])
                n335 = global read "Global Variables.vi" "zIris"() -> (w589:dbl[])
                n336 = call-poly <vilib>:"Plot Helper.vi"("Plot ID"=6, "z vector"=w589, "y vector"=w590, "x vector"=w591, "3D Plot lvclass Array in"=w587) -> ("3D Plot lvclass Array out"=w586:refnum<class "3D Plot Datatype.lvclass">[])  [unwired: 1 in, 5 out]
              }
              frame Enabled {
              }
            }
            n337 = Index Array(array=w563) -> (element #1=w574:dbl, element #2=w573:dbl, element #3=w572:dbl)  [unwired: 3 in]
            n338 = Build Array (concatenate)(w571, w574) -> (w566:dbl[])
            n339 = Build Array (concatenate)(w570, w573) -> (w565:dbl[])
            n340 = Build Array (concatenate)(w569, w572) -> (w564:dbl[])
            n341 = call-poly <vilib>:"Plot Helper.vi"("Plot ID"=5, "z vector"=w564, "y vector"=w565, "x vector"=w566, "3D Plot lvclass Array in"=w550) -> ("3D Plot lvclass Array out"=w557:refnum<class "3D Plot Datatype.lvclass">[])  [unwired: 1 in, 5 out]
            n342 = call-poly <vilib>:"Plot Helper.vi"("Plot ID"=6, "z vector"=w569, "y vector"=w570, "x vector"=w571, "3D Plot lvclass Array in"=w557) -> ("3D Plot lvclass Array out"=→"Robot XYZ":refnum<class "3D Plot Datatype.lvclass">[])  [unwired: 1 in, 5 out]
          }
        }
        n343 = local read "Current System State"() -> (w530:T9)
        n344 = disable-structure shown="Disabled" {
          disable-tunnel: w532 -> [w596 _]
          disable-tunnel: [w595 _] -> w531
          disable-tunnel: w530 -> [w594 _]
          frame Disabled {
            # "Disable write to mitigate finished late"
            n345 = local read "Online Eye Model"() -> (w593:T1)
            n346 = call "WriteLog.vi"("Online Eye Model"=w593, "Current System State"=w594, "File In"=w596) -> ("File Out"=w595:refnum<file>)  [unwired: 8 in]
          }
          frame Enabled {
          }
        }
        n347 = local read "Program Stop"() -> (w542:bool)
        n348 = shared-variable "PXI-Robot\\JointAngles.lvlib\\SystemState"(w530) -> ()  [unwired: 1 in, 1 out]
      }
      n349 = while {
        shift-right: [w635] -> _
        shift-left: w86 -> [w636]
        shift-right: [w632] -> _
        shift-left: _ -> [w630]
        shift-right: [w631] -> _
        shift-left: _ -> [w629]
        stop <- "Program Stop" stop-if-true
        # "Control and State Logic Loop"
        n350 = Wait (ms)(milliseconds to wait=u32 50) -> ()  [unwired: 1 out]
        n351 = case shown="\"M/S Operation\"" w636 {
          selector: w636 -> [w752 w758 w780 w854 w874 w900 w909 w940 w980 w1008]
          tunnel: [w751 w759 w779 w853 w875 w901 w910 w941 w981 w1009] -> w635
          frame "Homing", Default {
            n352 = global read "Global Variables.vi" "state flag array"() -> (w753:bool[])
            n353 = Index Array(array=w753, index=0) -> (element=w750:bool)
            n354 = case shown="True" w750 {
              tunnel: [w755 w756] -> w751
              tunnel: w752 -> [w755 _]
              frame False {
                # "homing in process"
              }
              frame True {
                w756 = T9."M/S Initialization" ("Current State")
                # "finish homing"
                n355 = global write "Global Variables.vi" "state changing"(TRUE ("state changing")) -> ()
                n356 = local write "Current System State"(w756) -> ()
              }
            }
          }
          frame "M/S Initialization" {
            n357 = global read "Global Variables.vi" "state flag array"() -> (w761:bool[])
            n358 = Index Array(array=w761, index=1) -> (element=w760:bool)
            n359 = case shown="False" w760 {
              tunnel: [w768 w770] -> w759
              tunnel: w758 -> [w768 _]
              frame False {
                n360 = property on="MS/Auto" class="Bool (strict)"("DisabledEnum"=T16."Disabled and Grayed Out" ("Disabled")) -> ()  [unwired: 2 in, 2 out]
                n361 = global read "Global Variables.vi" "L1 to L3 M/S cmd"() -> (w767:dbl[])
                n362 = Index Array(array=w767) -> (element #1=w766:dbl, element #2=w765:dbl, element #3=w764:dbl, element #4=w763:dbl)  [unwired: 4 in]
                n363 = local write "L1 [deg]"(w766) -> ()
                n364 = local write "L2 [deg]"(w765) -> ()
                n365 = local write "L3 [mm]"(w764) -> ()
                n366 = local write "L4 [deg]"(w763) -> ()
              }
              frame True {
                w770 = T9."M/S Operation" ("Current State")
                n367 = global write "Global Variables.vi" "state changing"(TRUE ("state changing")) -> ()
                n368 = property on="MS/Auto" class="Bool (strict)"("DisabledEnum"=T16."Enabled" ("Disabled")) -> ()  [unwired: 2 in, 2 out]
                n369 = local write "Current System State"(w770) -> ()
              }
            }
          }
          frame "M/S Operation" {
            n370 = local read "MS/Auto"() -> (w778:bool)
            n371 = local read "Load Traj"() -> (w776:bool)
            n372 = Not(x=w778) -> (.not. x?=w777:bool)
            n373 = Build Array(w777, w776, "Home") -> (w775:bool[])
            n374 = Boolean Array To Number(Boolean array=w775) -> (number=w774:u32)
            n375 = case shown="0, Default" w774 {
              tunnel: w780 -> [w783 _ w844 _]
              tunnel: [w783 w840 w845 w852] -> w779
              frame 0, Default {
                n376 = global read "Global Variables.vi" "remote ctrl source"() -> (w782:u16)
                n377 = global write "Global Variables.vi" "irrigate"("Irrigation") -> ()
                n378 = case shown="1" w782 {
                  frame 0, Default {
                    n379 = Build Array("L1 [deg]", "L2 [deg]", "L3 [mm]") -> (w789:dbl[])
                    n380 = Build Array (concatenate)(w789, "L4 [deg]") -> (w790:dbl[])
                    n381 = global write "Global Variables.vi" "OCT Z cmd Posit"("OCT Cmd Z [mm]") -> ()
                    n382 = shared-variable "PXI-Robot\\JointAngles.lvlib\\L1 to L4 Cmd"(w790) -> ()  [unwired: 1 in, 1 out]
                    n383 = global write "Global Variables.vi" "L1 to L3 M/S cmd"(w789) -> ()
                    n384 = global write "Global Variables.vi" "L4 M/S cmd"("L4 [deg]") -> ()
                    n385 = Build Array("Stage Z [mm]", "Stage Y [mm]", "Stage X [mm]") -> (w786:dbl[])
                    n386 = global write "Global Variables.vi" "Stage cmd Posit"(w786) -> ()
                  }
                  frame 1 {
                    n387 = flat-sequence {
                      frame #0 {
                        # "Receive command from the cockpit"
                        n388 = local read "Tip out Posit"() -> (w798:dbl[])
                        n389 = local read "deltaXYZ"() -> (w797:sgl[])
                        n390 = local read "deltaRoll"() -> (w796:sgl)
                        n391 = call "Cockpit Cmd Inc.vi"("Tip out Posit"=w798, "deltaRoll"=w796, "deltaXYZ"=w797) -> ("Roll Out"=w799:sgl, "Z Out"=w800:sgl, "Y Out"=w801:sgl, "X Out"=w802:sgl)  [unwired: 5 in]
                        n392 = global read "Global Variables.vi" "armID"() -> (w807:i32)
                        n393 = call "Inverse Kinematics.vi"("isToolTipInsideEye"=TRUE, "armID"=w807, "z"=w800, "y"=w801, "x"=w802) -> ("j3"=w803:dbl, "j2"=w804:dbl, "j1"=w805:dbl)  [unwired: 3 in, 1 out]
                        n394 = Build Array(w805, w804, w803) -> (w806:dbl[])
                        n395 = global write "Global Variables.vi" "L1 to L3 M/S cmd"(w806) -> ()
                        n396 = global write "Global Variables.vi" "L4 M/S cmd"(w799) -> ()
                      }
                      frame #1 {
                        # "Send current robot readings"
                        n397 = disable-structure shown="Disabled" {
                          frame Disabled {
                            n398 = local read "Tip out Posit"() -> (w809:dbl[])
                            n399 = local read "Grasp out"() -> (w814:dbl)
                            n400 = local read item#-1() -> (w813)
                            n401 = Index Array(array=w809) -> (element #1=w810:dbl, element #2=w811:dbl, element #3=w812:dbl)  [unwired: 3 in]
                            n402 = call "Cockpit UDP Sender IRISSv2.vi"("actual_gripper"=w814, "actual_rotation"=w813, "actual_Z"=w812, "actual_Y"=w811, "actual_X"=w810) -> ()  [unwired: 7 in]
                          }
                          frame Enabled {
                          }
                        }
                      }
                    }
                    n403 = local read "OCT Cmd Z [mm]"() -> (w795:dbl)
                    n404 = global write "Global Variables.vi" "OCT Z cmd Posit"(w795) -> ()
                  }
                  frame 2 {
                    n405 = shared-variable "PXI-Robot\\JointAngles.lvlib\\StagePosition - X"() -> (w817:dbl)  [unwired: 1 in, 1 out]
                    n406 = shared-variable "PXI-Robot\\JointAngles.lvlib\\StagePosition - Y"() -> (w816:dbl)  [unwired: 1 in, 1 out]
                    n407 = shared-variable "PXI-Robot\\JointAngles.lvlib\\StagePosition - Z"() -> (w815:dbl)  [unwired: 1 in, 1 out]
                    n408 = shared-variable "PXI-Robot\\JointAngles.lvlib\\OCT z command"() -> (w821:dbl)  [unwired: 1 in, 1 out]
                    n409 = local write "OCT Cmd Z [mm]"(w821) -> ()
                    n410 = local write "Stage Z [mm]"(w817) -> ()
                    n411 = local write "Stage Y [mm]"(w816) -> ()
                    n412 = local write "Stage X [mm]"(w815) -> ()
                    n413 = shared-variable "PXI-Robot\\JointAngles.lvlib\\Move XYZ"() -> (w819:bool)  [unwired: 1 in, 1 out]
                    n414 = global read "Global Variables.vi" "Inside RCM"() -> (w818:bool)
                    n415 = And(x=w819, y=w818) -> (x .and. y?=w820:bool)
                    n416 = case shown="False" w820 {
                      frame False {
                        n417 = shared-variable "PXI-Robot\\JointAngles.lvlib\\L1 to L4 Cmd"() -> (w827:dbl[])  [unwired: 1 in, 1 out]
                        n418 = Index Array(array=w827) -> (element #1=w824:dbl, element #2=w823:dbl, element #3=w822:dbl, element #4=w826:dbl)  [unwired: 4 in]
                        n419 = local write "L4 [deg]"(w826) -> ()
                        n420 = global write "Global Variables.vi" "L4 M/S cmd"(w826) -> ()
                        n421 = Build Array(w824, w823, w822) -> (w825:dbl[])
                        n422 = global write "Global Variables.vi" "L1 to L3 M/S cmd"(w825) -> ()
                        n423 = local write "L3 [mm]"(w822) -> ()
                        n424 = local write "L1 [deg]"(w824) -> ()
                        n425 = local write "L2 [deg]"(w823) -> ()
                      }
                      frame True {
                        w831 = 0.0 ("element")
                        n426 = shared-variable "PXI-Robot\\JointAngles.lvlib\\XYZ Cmd"() -> (w835:dbl[])  [unwired: 1 in, 1 out]
                        n427 = global read "Global Variables.vi" "armID"() -> (w834:i32)
                        n428 = Index Array(array=w835) -> (element #1=w838:dbl, element #2=w837:dbl, element #3=w836:dbl)  [unwired: 3 in]
                        n429 = call "Inverse Kinematics.vi"("isToolTipInsideEye"=TRUE, "armID"=w834, "z"=w836, "y"=w837, "x"=w838) -> ("j3"=w830:dbl, "j2"=w829:dbl, "j1"=w828:dbl)  [unwired: 3 in, 1 out]
                        n430 = Build Array(w828, w829, w830) -> (w832:dbl[])
                        n431 = Build Array(w828, w829, w830, w831) -> (w833:dbl[])
                        n432 = global write "Global Variables.vi" "L1 to L3 M/S cmd"(w832) -> ()
                        n433 = shared-variable "PXI-Robot\\JointAngles.lvlib\\L1 to L4 Cmd"(w833) -> ()  [unwired: 1 in, 1 out]
                        n434 = global write "Global Variables.vi" "L4 M/S cmd"(w831) -> ()
                      }
                    }
                  }
                }
              }
              frame 1 {
                w840 = T9."Aiming" ("Current State")
                n435 = global write "Global Variables.vi" "state changing"(TRUE ("state changing")) -> ()
                n436 = local write "Current System State"(w840) -> ()
                n437 = property on="MS/Auto" class="Bool (strict)"("DisabledEnum"=T16."Disabled and Grayed Out" ("Disabled")) -> ()  [unwired: 2 in, 2 out]
              }
              frame 2 {
                n438 = global read "Global Variables.vi" "Inside RCM"() -> (w843:bool)
                n439 = case shown="True" w843 {
                  tunnel: [w846 w847] -> w845
                  tunnel: w844 -> [w846 _]
                  frame False {
                  }
                  frame True {
                    w847 = T9."Trajectory Loading" ("Current State")
                    w848 = FALSE ("MS/Auto")
                    n440 = global write "Global Variables.vi" "state changing"(TRUE ("state changing")) -> ()
                    n441 = local write "MS/Auto"(w848) -> ()
                    n442 = local write "Load Traj"(w848) -> ()
                    n443 = local write "Current System State"(w847) -> ()
                    n444 = property on="MS/Auto" class="Bool (strict)"("DisabledEnum"=T16."Disabled and Grayed Out" ("Disabled")) -> ()  [unwired: 2 in, 2 out]
                  }
                }
              }
              frame 4 {
                w852 = T9."Homing" ("Current State")
                w851 = TRUE ("state changing")
                n445 = global write "Global Variables.vi" "state changing"(w851) -> ()
                n446 = global write "Global Variables.vi" "Enforce Homing"(w851) -> ()
                n447 = local write "Current System State"(w852) -> ()
              }
            }
          }
          frame "Aiming" {
            n448 = global read "Global Variables.vi" "state flag array"() -> (w856:bool[])
            n449 = Index Array(array=w856, index=3) -> (element=w855:bool)
            n450 = case shown="True" w855 {
              tunnel: w854 -> [w858 w862]
              tunnel: [w858 w861] -> w853
              frame False {
              }
              frame True {
                n451 = property on="MS/Auto" class="Bool (strict)"("DisabledEnum"=T16."Enabled" ("Disabled")) -> ()  [unwired: 2 in, 2 out]
                n452 = Build Array("Insert", "MS/Auto") -> (w866:bool[])
                n453 = Boolean Array To Number(Boolean array=w866) -> (number=w863:u32)
                n454 = case shown="1" w863 {
                  tunnel: w862 -> [w867 _ _]
                  tunnel: [w867 w868 w872] -> w861
                  frame 0, Default {
                  }
                  frame 1 {
                    w868 = T9."Engaging" ("Current State")
                    n455 = global write "Global Variables.vi" "state changing"(TRUE ("state changing")) -> ()
                    n456 = local write "Insert"(FALSE ("Enter")) -> ()
                    n457 = property on="MS/Auto" class="Bool (strict)"("DisabledEnum"=T16."Disabled and Grayed Out" ("Disabled")) -> ()  [unwired: 2 in, 2 out]
                    n458 = local write "Current System State"(w868) -> ()
                  }
                  frame 2 {
                    w872 = T9."M/S Initialization" ("Current State")
                    n459 = global write "Global Variables.vi" "state changing"(TRUE ("state changing")) -> ()
                    n460 = local write "Current System State"(w872) -> ()
                  }
                }
                n461 = local read "OCT Cmd Z [mm]"() -> (w859:dbl)
                n462 = global write "Global Variables.vi" "OCT Z cmd Posit"(w859) -> ()
              }
            }
          }
          frame "Engaging" {
            n463 = global read "Global Variables.vi" "state flag array"() -> (w877:bool[])
            n464 = Index Array(array=w877, index=4) -> (element=w876:bool)
            n465 = case shown="True" w876 {
              tunnel: [w880 w887] -> w875
              tunnel: w874 -> [w881 w888]
              frame False {
                n466 = local read "Retract"() -> (w879:bool)
                n467 = case shown="False" w879 {
                  tunnel: [w882 w883] -> w880
                  tunnel: w881 -> [w882 _]
                  frame False {
                  }
                  frame True {
                    w883 = T9."Aiming" ("Current State")
                    n468 = global write "Global Variables.vi" "state changing"(TRUE ("state changing")) -> ()
                    n469 = local write "Retract"(FALSE ("Retract")) -> ()
                    n470 = local write "Current System State"(w883) -> ()
                  }
                }
              }
              frame True {
                n471 = Build Array("Load Traj", "Retract") -> (w891:bool[])
                n472 = Boolean Array To Number(Boolean array=w891) -> (number=w889:u32)
                n473 = case shown="2" w889 {
                  tunnel: w888 -> [w892 _ _]
                  tunnel: [w892 w893 w896] -> w887
                  frame 0, Default {
                  }
                  frame 1 {
                    w893 = T9."Trajectory Loading" ("Current State")
                    n474 = global write "Global Variables.vi" "state changing"(TRUE ("state changing")) -> ()
                    n475 = local write "Load Traj"(FALSE ("Load Traj")) -> ()
                    n476 = local write "Current System State"(w893) -> ()
                  }
                  frame 2 {
                    w896 = T9."Aiming" ("Current State")
                    n477 = global write "Global Variables.vi" "state changing"(TRUE ("state changing")) -> ()
                    n478 = local write "Retract"(FALSE ("Load Traj")) -> ()
                    n479 = local write "Current System State"(w896) -> ()
                  }
                }
              }
            }
          }
          frame "Trajectory Loading" {
            n480 = global read "Global Variables.vi" "state flag array"() -> (w903:bool[])
            n481 = global write "Global Variables.vi" "irrigate"(TRUE ("irrigate")) -> ()
            n482 = Index Array(array=w903, index=2) -> (element=w902:bool)
            n483 = case shown="True" w902 {
              tunnel: [w905 w906] -> w901
              tunnel: w900 -> [w905 _]
              frame False {
              }
              frame True {
                w906 = T9."Tracking Initialization" ("Current State")
                n484 = global write "Global Variables.vi" "state changing"(TRUE ("state changing")) -> ()
                n485 = local write "Current System State"(w906) -> ()
              }
            }
          }
          frame "Tracking Initialization" {
            n486 = global read "Global Variables.vi" "state flag array"() -> (w912:bool[])
            n487 = Index Array(array=w912, index=5) -> (element=w911:bool)
            n488 = case shown="True" w911 {
              tunnel: [w914 w921] -> w910
              tunnel: w909 -> [w914 w920]
              frame False {
              }
              frame True {
                n489 = local read "Load Traj"() -> (w922:bool)
                n490 = local read "Retract"() -> (w916:bool)
                n491 = local read "To Regulation"() -> (w915:bool)
                n492 = Or(x="Initialize", y=w916) -> (x .or. y?=w918:bool)
                n493 = Build Array("Track", w922, w918, w915) -> (w924:bool[])
                n494 = Boolean Array To Number(Boolean array=w924) -> (number=w923:u32)
                n495 = case shown="1" w923 {
                  tunnel: [w925 w926 w929 w932 w935] -> w921
                  tunnel: w920 -> [w925 _ _ _ _]
                  frame 0, Default {
                  }
                  frame 1 {
                    w926 = T9."Tracking" ("Current State")
                    n496 = global write "Global Variables.vi" "state changing"(TRUE ("state changing")) -> ()
                    n497 = local write "Track"(FALSE ("Track")) -> ()
                    n498 = local write "Current System State"(w926) -> ()
                  }
                  frame 2 {
                    w929 = T9."Trajectory Loading" ("Current State")
                    n499 = global write "Global Variables.vi" "state changing"(TRUE ("state changing")) -> ()
                    n500 = local write "Load Traj"(FALSE ("Load Traj")) -> ()
                    n501 = local write "Current System State"(w929) -> ()
                  }
                  frame 4 {
                    w932 = T9."Engaging" ("Current State")
                    n502 = global write "Global Variables.vi" "state changing"(TRUE ("state changing")) -> ()
                    n503 = local write "Initialize"(FALSE ("Load Traj")) -> ()
                    n504 = local write "Current System State"(w932) -> ()
                  }
                  frame 8 {
                    w935 = T9."Tracking" ("Current State")
                    w936 = FALSE  # Reset
                    n505 = global write "Global Variables.vi" "state changing"(TRUE ("state changing")) -> ()
                    n506 = local write "Track"(FALSE ("Track")) -> ()
                    n507 = local write "Current System State"(w935) -> ()
                    n508 = local write "To Regulation"(w936) -> ()
                  }
                }
              }
            }
            n509 = global write "Global Variables.vi" "irrigate"(TRUE ("irrigate")) -> ()
          }
          frame "Tracking" {
            n510 = global read "Global Variables.vi" "state flag array"() -> (w943:bool[])
            n511 = Index Array(array=w943, index=6) -> (element=w942:bool)
            n512 = case shown="True" w942 {
              tunnel: [w945 w963] -> w941
              tunnel: w940 -> [w945 w962]
              frame False {
              }
              frame True {
                (unwired) 90 ("y")
                n513 = local read "Initialize"() -> (w959:bool)
                n514 = local read "Retract"() -> (w956:bool)
                n515 = local read "Go to Assign Pt"() -> (w957:bool)
                n516 = local read "To Regulation"() -> (w958:bool)
                n517 = local read "Timer"() -> (w955:i32)
                n518 = local read "Total Time"() -> (w946:i16)
                n519 = global write "Global Variables.vi" "irrigate"(TRUE ("irrigate")) -> ()
                n520 = Quotient & Remainder(x=w955, y=w946) -> (x-y*floor(x/y)=w954:i32, floor(x/y)=w949:i32)
                n521 = Equal To 0?(x=w954) -> (x = 0?=w953:bool)
                n522 = Not Equal To 0?(x=w949) -> (x != 0?=w948:bool)
                n523 = call "RisingEdge.vi"("Signal In"=w953) -> ("Rising Edge"=w952:bool)  [unwired: 10 in]
                n524 = Compound Arithmetic op=AND(w952, w948, "Stop-and-Go") -> (w951:bool)
                n525 = Build Array(w959, w956, w957, w958, w951) -> (w961:bool[])
                n526 = Boolean Array To Number(Boolean array=w961) -> (number=w960:u32)
                n527 = case shown="4" w960 {
                  tunnel: [w964 w965 w968 w971 w974 w976] -> w963
                  tunnel: w962 -> [w964 _ _ _ _ _]
                  frame 0, Default {
                  }
                  frame 1 {
                    w965 = T9."Engaging" ("Current State")
                    n528 = global write "Global Variables.vi" "state changing"(TRUE ("state changing")) -> ()
                    n529 = local write "Initialize"(FALSE ("Load Traj")) -> ()
                    n530 = local write "Current System State"(w965) -> ()
                  }
                  frame 2 {
                    w968 = T9."Aiming" ("Current State")
                    n531 = global write "Global Variables.vi" "state changing"(TRUE ("state changing")) -> ()
                    n532 = local write "Retract"(FALSE ("Load Traj")) -> ()
                    n533 = local write "Current System State"(w968) -> ()
                  }
                  frame 4 {
                    w971 = T9."Rerouting" ("Current State")
                    n534 = global write "Global Variables.vi" "state changing"(TRUE ("state changing")) -> ()
                    n535 = local write "Go to Assign Pt"(FALSE ("Load Traj")) -> ()
                    n536 = local write "Current System State"(w971) -> ()
                  }
                  frame 8 {
                    w974 = T9."Regulation" ("Current State")
                    n537 = global write "Global Variables.vi" "state changing"(TRUE ("state changing")) -> ()
                    n538 = local write "Current System State"(w974) -> ()
                  }
                  frame 16 {
                    w976 = T9."Regulation" ("Current State")
                    n539 = global write "Global Variables.vi" "state changing"(TRUE ("state changing")) -> ()
                    n540 = local write "To Regulation"(TRUE ("state changing")) -> ()
                    n541 = local write "Current System State"(w976) -> ()
                  }
                }
              }
            }
            n542 = global write "Global Variables.vi" "irrigate"(TRUE ("irrigate")) -> ()
          }
          frame "Rerouting" {
            n543 = global read "Global Variables.vi" "state flag array"() -> (w983:bool[])
            n544 = Index Array(array=w983, index=7) -> (element=w982:bool)
            n545 = case shown="True" w982 {
              tunnel: [w987 w1001] -> w981
              tunnel: w980 -> [w986 _]
              frame False {
                n546 = shared-variable "PXI-Robot\\JointAngles.lvlib\\EmergencyAlarmBit"() -> (w993:bool)  [unwired: 1 in, 1 out]
                n547 = local read "Initialize"() -> (w992:bool)
                n548 = local read "Retract"() -> (w985:bool)
                n549 = local read "Go to Assign Pt"() -> (w989:bool)
                n550 = Compound Arithmetic op=OR(w993, w992, w985) -> (w990:bool)
                n551 = Build Array(w990, w989) -> (w991:bool[])
                n552 = Boolean Array To Number(Boolean array=w991) -> (number=w988:u32)
                n553 = case shown="2" w988 {
                  tunnel: w986 -> [w994 _ _]
                  tunnel: [w994 w995 w998] -> w987
                  frame 0, Default {
                  }
                  frame 1 {
                    w995 = T9."Engaging" ("Current State")
                    n554 = global write "Global Variables.vi" "state changing"(TRUE ("state changing")) -> ()
                    n555 = local write "Initialize"(FALSE ("Initialize")) -> ()
                    n556 = local write "Current System State"(w995) -> ()
                  }
                  frame 2 {
                    w998 = T9."Rerouting" ("Current State")
                    n557 = global write "Global Variables.vi" "state changing"(TRUE ("state changing")) -> ()
                    n558 = local write "Go to Assign Pt"(FALSE ("Initialize")) -> ()
                    n559 = local write "Current System State"(w998) -> ()
                  }
                }
              }
              frame True {
                n560 = local read "To Regulation"() -> (w1002:bool)
                n561 = case shown="False" w1002 {
                  tunnel: [T9."Tracking" ("Current State") T9."Regulation" ("Current State")] -> w1001
                  frame False {
                    n562 = global write "Global Variables.vi" "state changing"(TRUE ("state changing")) -> ()
                  }
                  frame True {
                    n563 = global write "Global Variables.vi" "state changing"(TRUE ("state changing")) -> ()
                  }
                }
                n564 = local write "Current System State"(w1001) -> ()
              }
            }
            n565 = global write "Global Variables.vi" "irrigate"(TRUE ("irrigate")) -> ()
          }
          frame "Regulation" {
            n566 = global read "Global Variables.vi" "state flag array"() -> (w1011:bool[])
            n567 = Index Array(array=w1011, index=8) -> (element=w1010:bool)
            n568 = case shown="True" w1010 {
              tunnel: [w1020 w1032] -> w1009
              tunnel: w1008 -> [w1019 w1033]
              frame False {
                n569 = local read "Initialize"() -> (w1018:bool)
                n570 = local read "Retract"() -> (w1017:bool)
                n571 = local read "Go to Assign Pt"() -> (w1013:bool)
                n572 = Or(x=w1018, y=w1017) -> (x .or. y?=w1016:bool)
                n573 = Build Array(w1016, w1013) -> (w1015:bool[])
                n574 = Boolean Array To Number(Boolean array=w1015) -> (number=w1014:u32)
                n575 = case shown="2" w1014 {
                  tunnel: w1019 -> [w1021 _ _]
                  tunnel: [w1021 w1023 w1026] -> w1020
                  frame 0, Default {
                  }
                  frame 1 {
                    w1022 = FALSE  # Reset
                    w1023 = T9."Engaging" ("Current State")
                    n576 = global write "Global Variables.vi" "state changing"(TRUE ("state changing")) -> ()
                    n577 = local write "Initialize"(FALSE ("Load Traj")) -> ()
                    n578 = local write "Current System State"(w1023) -> ()
                    n579 = local write "To Regulation"(w1022) -> ()
                  }
                  frame 2 {
                    w1026 = T9."Rerouting" ("Current State")
                    n580 = global write "Global Variables.vi" "state changing"(TRUE ("state changing")) -> ()
                    n581 = local write "Go to Assign Pt"(FALSE ("Initialize")) -> ()
                    n582 = local write "Current System State"(w1026) -> ()
                  }
                }
              }
              frame True {
                n583 = local read "Load Traj"() -> (w1035:bool)
                n584 = local read "Go to Assign Pt"() -> (w1036:bool)
                n585 = local read "Initialize"() -> (w1031:bool)
                n586 = local read "Retract"() -> (w1029:bool)
                n587 = local read "Track"() -> (w1030:bool)
                n588 = Build Array(w1035, w1036, w1031, w1029, w1030) -> (w1037:bool[])
                n589 = Boolean Array To Number(Boolean array=w1037) -> (number=w1034:u32)
                n590 = case shown="2" w1034 {
                  tunnel: w1033 -> [w1038 _ _ _ _ _]
                  tunnel: [w1038 w1040 w1043 w1047 w1051 w1055] -> w1032
                  frame 0, Default {
                  }
                  frame 1 {
                    w1039 = FALSE  # Reset
                    w1040 = T9."Trajectory Loading" ("Current State")
                    n591 = global write "Global Variables.vi" "state changing"(TRUE ("state changing")) -> ()
                    n592 = local write "Load Traj"(FALSE ("Load Traj")) -> ()
                    n593 = local write "Current System State"(w1040) -> ()
                    n594 = local write "To Regulation"(w1039) -> ()
                  }
                  frame 2 {
                    w1043 = T9."Rerouting" ("Current State")
                    n595 = global write "Global Variables.vi" "state changing"(TRUE ("state changing")) -> ()
                    n596 = local write "Go to Assign Pt"(FALSE ("Load Traj")) -> ()
                    n597 = local write "Current System State"(w1043) -> ()
                  }
                  frame 4 {
                    w1046 = FALSE  # Reset
                    w1047 = T9."Engaging" ("Current State")
                    n598 = global write "Global Variables.vi" "state changing"(TRUE ("state changing")) -> ()
                    n599 = local write "Initialize"(FALSE ("Load Traj")) -> ()
                    n600 = local write "To Regulation"(w1046) -> ()
                    n601 = local write "Current System State"(w1047) -> ()
                  }
                  frame 8 {
                    w1050 = FALSE  # Reset
                    w1051 = T9."Aiming" ("Current State")
                    n602 = global write "Global Variables.vi" "state changing"(TRUE ("state changing")) -> ()
                    n603 = local write "Retract"(FALSE ("Load Traj")) -> ()
                    n604 = local write "To Regulation"(w1050) -> ()
                    n605 = local write "Current System State"(w1051) -> ()
                  }
                  frame 16 {
                    w1054 = FALSE  # Reset
                    w1055 = T9."Tracking" ("Current State")
                    n606 = global write "Global Variables.vi" "state changing"(TRUE ("state changing")) -> ()
                    n607 = local write "Track"(FALSE ("Load Traj")) -> ()
                    n608 = local write "Current System State"(w1055) -> ()
                    n609 = local write "To Regulation"(w1054) -> ()
                  }
                }
              }
            }
            n610 = global write "Global Variables.vi" "irrigate"(TRUE ("irrigate")) -> ()
          }
        }
        n611 = flat-sequence {
          tunnel: [w649] -> w621
          tunnel: [w648] -> w620
          tunnel: w630 -> [w647]
          tunnel: w629 -> [w646]
          tunnel: w621 -> [w677]
          tunnel: w620 -> [w676]
          tunnel: [w677] -> w619
          tunnel: [w676] -> w618
          tunnel: w619 -> [w705]
          tunnel: [w705] -> w617
          tunnel: w618 -> [w722]
          tunnel: [w722] -> w616
          tunnel: [w735] -> w615
          tunnel: w617 -> [w745]
          tunnel: [w745] -> w614
          tunnel: w616 -> [w735]
          tunnel: [w749] -> w631
          tunnel: w615 -> [w749]
          tunnel: [w748] -> w632
          tunnel: w614 -> [w748]
          frame #0 {
            # "Check if Trajectory is (Re)loaded"
            n612 = local read "Update Mdl & Traj"() -> (w651:bool)
            n613 = call "RisingEdge.vi"("Signal In"=w651) -> ("Rising Edge"=w650:bool)  [unwired: 10 in]
            n614 = case shown="True" w650 {
              tunnel: [w652 w673] -> w648
              tunnel: [w653 w662] -> w649
              tunnel: w647 -> [w653 _]
              tunnel: w646 -> [w652 _]
              frame False {
                # "Use Nominal Model & Trajectory"
              }
              frame True {
                w655 = u16 3 items=["4x", "3x", "2x", "1x", "0.5x", "0.2x", "0.1x", "PAUSE"] ("Speed Override")
                w667 = 2 ("index")
                # "Update Trajectory and Model after \"Trajectory Loading\""
                n615 = local read "Trajectory Cluster"() -> (w662:T2)
                n616 = local read "Eye Model Cluster"() -> (w660:T4)
                n617 = local write "Update Mdl & Traj"(FALSE ("Update Model")) -> ()
                n618 = global write "Global Variables.vi" "current run no."(u8 1 ("current run no.")) -> ()
                n619 = local write "Speed Override"(w655) -> ()
                n620 = Unbundle By Name(w662) -> ("Depth Array"=w664:dbl[])
                n621 = shared-variable "PXI-Robot\\JointAngles.lvlib\\Offline Eye Model"(w660) -> ()  [unwired: 1 in, 1 out]
                n622 = call "Extract Depth Param.vi"("Eye Model Cluster"=w660) -> ("Nominal Model param"=w673:T19)
                n623 = Unbundle By Name(w660) -> ("za_true"=w672:dbl, "za_work"=w671:dbl, "zp_work"=→"PO Cruising":dbl, "zp_true"=w669:dbl, "Iris Center"=w666:dbl[])
                n624 = Array Size(array=w664) -> (size(s)=→"No. of Runs":i32)
                n625 = Index Array(array=w666, index=w667) -> (element=w670:dbl)
                n626 = Array Subset(array=w666, index=0, length=w667) -> (w665:dbl[])
                n627 = local write "Iris XY Scaling"(dbl[] [1.0, 1.0]) -> ()
                n628 = local write "Depth Offset"(0.0 ("Depth Offset")) -> ()
                n629 = local write "Rotation"(dbl[] [0.0, 0.0, 0.0]) -> ()
                n630 = local write "PO No-Fly"(w669) -> ()
                n631 = local write "AN No-Fly"(w672) -> ()
                n632 = local write "AN Cruising"(w671) -> ()
                n633 = local write "Iris XY Center"(w665) -> ()
                n634 = local write "Iris Center"(w670) -> ()
              }
            }
          }
          frame #1 {
            # "Update Working Depth After Each Cycle"
            n635 = shared-variable "PXI-Robot\\JointAngles.lvlib\\RemoteSenderEngaged"() -> (w674:bool)  [unwired: 1 in, 1 out]
            n636 = case shown="True" w674 {
              frame False {
                n637 = global write "Global Variables.vi" "assign pt (x,y,z)"("Assign Point [mm]") -> ()
                n638 = global write "Global Variables.vi" "max limit [mmHg]"("Max Limit [mmHg]") -> ()
                n639 = global write "Global Variables.vi" "speed override"("Speed Override") -> ()
              }
              frame True {
                w681 = u16 2 items=["None", "Surgical Console", "Joystick", "MJG Teleoperation", "MJG C++ Teleoperation"] ("Remote Control Source 2")
                w686 = 2 ("index")
                n640 = shared-variable "PXI-Robot\\JointAngles.lvlib\\EmergencyAlarmBit"() -> (w698:bool)  [unwired: 1 in, 1 out]
                n641 = shared-variable "PXI-Robot\\JointAngles.lvlib\\Go 2 Assign Point"() -> (w695:bool)  [unwired: 1 in, 1 out]
                n642 = shared-variable "PXI-Robot\\JointAngles.lvlib\\Online Eye Model"() -> (w691:T20)  [unwired: 1 in, 1 out]
                n643 = global write "Global Variables.vi" "remote ctrl source"(w681) -> ()
                n644 = local write "Remote Control Source"(w681) -> ()
                n645 = Unbundle By Name(w691) -> ("za_true"=w694:dbl, "za_work"=w693:dbl, "zp_true"=w692:dbl, "Iris Center"=w683:dbl[])
                n646 = call "RisingEdge.vi"("Signal In"=w698) -> ("Rising Edge"=w697:bool)  [unwired: 10 in]
                n647 = call "RisingEdge.vi"("Signal In"=w695) -> ("Rising Edge"=w696:bool)  [unwired: 10 in]
                n648 = Index Array(array=w683, index=w686) -> (element=w684:dbl)
                n649 = Array Subset(array=w683, index=0, length=w686) -> (w687:dbl[])
                n650 = case shown="True" w697 {
                  selector: w697 -> [_ w701]
                  frame False {
                  }
                  frame True {
                    n651 = local write "L3 Go Home"(w701) -> ()
                  }
                }
                n652 = local write "Go to Assign Pt"(w696) -> ()
                n653 = local write "AN No-Fly"(w694) -> ()
                n654 = local write "AN Cruising"(w693) -> ()
                n655 = local write "PO No-Fly"(w692) -> ()
                n656 = local write "Iris XY Center"(w687) -> ()
                n657 = local write "Iris Center"(w684) -> ()
                n658 = shared-variable "PXI-Robot\\JointAngles.lvlib\\Assign Point"() -> (w699:dbl[])  [unwired: 1 in, 1 out]
                n659 = shared-variable "PXI-Robot\\JointAngles.lvlib\\Max Vacuum"() -> (w682:dbl)  [unwired: 1 in, 1 out]
                n660 = shared-variable "PXI-Robot\\JointAngles.lvlib\\Depth Offset"() -> (w690:dbl)  [unwired: 1 in, 1 out]
                n661 = shared-variable "PXI-Robot\\JointAngles.lvlib\\Iris XY Scaling"() -> (w689:dbl[])  [unwired: 1 in, 1 out]
                n662 = shared-variable "PXI-Robot\\JointAngles.lvlib\\DeformArrayRot"() -> (w688:dbl[])  [unwired: 1 in, 1 out]
                n663 = shared-variable "PXI-Robot\\JointAngles.lvlib\\Track Speed"() -> (w700:u16)  [unwired: 1 in, 1 out]
                n664 = global write "Global Variables.vi" "max limit [mmHg]"(w682) -> ()
                n665 = local write "Max Limit [mmHg]"(w682) -> ()
                n666 = local write "Assign Point [mm]"(w699) -> ()
                n667 = global write "Global Variables.vi" "assign pt (x,y,z)"(w699) -> ()
                n668 = global write "Global Variables.vi" "speed override"(w700) -> ()
                n669 = local write "Speed Override"(w700) -> ()
                n670 = local write "Iris XY Scaling"(w689) -> ()
                n671 = local write "Depth Offset"(w690) -> ()
                n672 = local write "Rotation"(w688) -> ()
              }
            }
            n673 = Not(x=w674) -> (.not. x?=w675:bool)
            n674 = global write "Global Variables.vi" "lock robot"(w675) -> ()
          }
          frame #2 {
            n675 = local read "PO No-Fly"() -> (w716:dbl)
            n676 = local read "Iris Center"() -> (w717:dbl)
            n677 = local read "Depth Offset"() -> (w721:dbl)
            n678 = global read "Global Variables.vi" "current run no."() -> (w714:u8)
            n679 = local read "Speed Override"() -> (w711:u16)
            n680 = Unbundle By Name(w705) -> ("Speed Array"=w713:dbl[])
            n681 = Unbundle By Name(w705) -> ("Depth Array"=w712:dbl[])
            n682 = Bundle By Name(cluster=cluster{"zi":dbl, "zp_true":dbl} {"zi"=0.0, "zp_true"=-2.5} ("z Cluster"), "zi"=w717, "zp_true"=w716) -> (w703:cluster{"zi":dbl, "zp_true":dbl})
            n683 = Increment(x=w714) -> (x+1=w715:u8)
            n684 = case shown="4" w711 {
              tunnel: [4.0 ("y") 3.0 ("y") 2.0 ("y") 1.0 ("y") 0.5 ("y") 0.2 ("y") 0.1 ("y") 0.0 ("y")] -> w708
              frame 0 {
                # "4X"
              }
              frame 1 {
                # "3X"
              }
              frame 2 {
                # "2X"
              }
              frame 3, Default {
                # "1x"
              }
              frame 4 {
                # "0.5x"
              }
              frame 5 {
                # "0.2x"
              }
              frame 6 {
                # "0.1x"
              }
              frame 7 {
                # "Pause"
              }
            }
            n685 = call "Depth Control.vi"("Current Run No."=w714, "Depth Offset"=w721, "Depth Array"=w712, "z Cluster"=w703) -> ("zp_work"=w702:dbl, "Schedule Depth & Speed"=w720:cluster{"Next Depth":dbl, "Current Depth":dbl})  [unwired: 6 in]
            n686 = call "Index Param Array.vi"("Index"=w714, "Array Input"=w713) -> ("Index Output"=w709:dbl)  [unwired: 9 in]
            n687 = call "Index Param Array.vi"("Index"=w715, "Array Input"=w713) -> ("Index Output"=w710:dbl)  [unwired: 9 in]
            n688 = Unbundle By Name(w720) -> ("Current Depth"=→"Current Depth":dbl, "Next Depth"=→"Next Depth":dbl)
            n689 = Multiply(x=w710, y=w708) -> (x*y=→"Next Speed":dbl)
            n690 = Multiply(x=w709, y=w708) -> (x*y=→"Current Speed":dbl)
            n691 = local write "PO Cruising"(w702) -> ()
            n692 = shared-variable "PXI-Robot\\JointAngles.lvlib\\PO_cruising"(w702) -> ()  [unwired: 1 in, 1 out]
            n693 = global write "Global Variables.vi" "speed schedule"(w710) -> ()
          }
          frame #3 {
            # "User High-Level Command Override"
            n694 = local read "PO Cruising"() -> (w737:dbl)
            n695 = Bundle By Name(cluster=T1 {"za_true"=0.0, "za_work"=0.0, "zi"=0.0, "zp_work"=0.0, "zp_true"=0.0, "Iris XY Center"=[0.0, 5.0], "Iris XY Scaling"=[1.0, 1.0]} ("High Level cmd"), "za_true"="AN No-Fly", "za_work"="AN Cruising", "zi"="Iris Center", "zp_work"=w737, "zp_true"="PO No-Fly", "Iris XY Center"="Iris XY Center", "Iris XY Scaling"="Iris XY Scaling") -> (w736:T1)
            "Online Eye Model" <- w736
            n696 = call "High Level Cmd Interpreter.vi"("Nominal Model param"=w735, "High Level cmd"=w736) -> ("Translation Array"=w732:dbl[], "Scaling Array"=w731:dbl[], "PC Displacement"=w733:dbl, "AC Displacement"=w734:dbl)  [unwired: 6 in]
            "Scaling" <- w731
            "Translation" <- w732
            n697 = global write "Global Variables.vi" "PC z displacement"(w733) -> ()
            n698 = global write "Global Variables.vi" "AC z displacement"(w734) -> ()
            n699 = Build Array (concatenate)(w731, "Rotation", w732) -> (w746:dbl[])
            n700 = global write "Global Variables.vi" "deform array"(w746) -> ()
          }
          frame #4 {
            # "Set/Reset Go to Assign Pt Flag"
          }
        }
        n701 = global write "Global Variables.vi" "increment ctrl"("Inc Ctrl") -> ()
        n702 = global write "Global Variables.vi" "z rot axis"("Z Rot Axis") -> ()
        n703 = global write "Global Variables.vi" "reroute transit vacf"("Reroute Transit Vacf") -> ()
        n704 = global write "Global Variables.vi" "vac extremum"("Vac Extremum") -> ()
        n705 = global write "Global Variables.vi" "z dist thld"("Z Dist Thld") -> ()
        n706 = global write "Global Variables.vi" "joint limits"("Joint Limits") -> ()
        n707 = global write "Global Variables.vi" "refractive index"("Refractive Index") -> ()
        n708 = global write "Global Variables.vi" "min AC gap"("Min AC Gap") -> ()
        n709 = global write "Global Variables.vi" "min PC gap"("Min PC Gap") -> ()
        n710 = global write "Global Variables.vi" "reroute hold [sec]"("Reroute Hold [sec]") -> ()
        n711 = global read "Global Variables.vi" "irrigate"() -> (w603:bool)
        n712 = call "RisingEdge.vi"("Signal In"="Go to Assign Pt") -> ("Rising Edge"=w622:bool)  [unwired: 10 in]
        n713 = Multiply(x="IV Height [mmHg]", y=1.36) -> (x*y=w599:dbl)
        n714 = global write "Global Variables.vi" "reset joystick"("Reset Joystick") -> ()
        n715 = global write "Global Variables.vi" "L3 go home"("L3 Go Home") -> ()
        n716 = global write "Global Variables.vi" "stop accurus"("Stop Accurus") -> ()
        n717 = global write "Global Variables.vi" "go to regulation"("To Regulation") -> ()
        n718 = global write "Global Variables.vi" "remote ctrl source"("Remote Control Source") -> ()
        n719 = local write "Go to Assign Pt"(w622) -> ()
        n720 = shared-variable "PXI-Robot\\JointAngles.lvlib\\Eye No"("Eye No") -> ()  [unwired: 1 in, 1 out]
        n721 = shared-variable "PXI-Robot\\JointAngles.lvlib\\Irrigation"(w603) -> ()  [unwired: 1 in, 1 out]
        n722 = To Long Integer(number=w599) -> (32bit integer=w600:i32)
        n723 = shared-variable "PXI-Robot\\JointAngles.lvlib\\Irrigation Height"(w600) -> ()  [unwired: 1 in, 1 out]
        n724 = global read "Global Variables.vi" "armID"() -> (w612:i32)
        n725 = call "RobotDll (SubVI).vi"("ArmPower"="Arm Power", "XYZ Stage Power"="XYZ Stage Power", "ArmID"=w612) -> ("ReceiveCount"=w611:u64, "SendCount"=w610:u64, "RobotConnection"=→"Status":bool)  [unwired: 10 in, 4 out]
        n726 = call "RobotDLLError(SubVI).vi"("ArmID"=w612) -> ("RobotStatusArray"=w608:bool[])  [unwired: 5 in, 9 out]
        n727 = global write "Global Variables.vi" "Robot Status Array"(w608) -> ()
        n728 = global write "Global Variables.vi" "Receive Count"(w611) -> ()
        n729 = global write "Global Variables.vi" "Send Count"(w610) -> ()
        n730 = Index Array(array=w608, index=6) -> (element=w606:bool)
        n731 = Not(x=w606) -> (.not. x?=w605:bool)
        n732 = global write "Global Variables.vi" "program stop"("Program Stop") -> ()
        n733 = shared-variable "PXI-Robot\\JointAngles.lvlib\\Inside RCM"(w605) -> ()  [unwired: 1 in, 1 out]
        n734 = global write "Global Variables.vi" "Inside RCM"(w605) -> ()
      }
      n735 = node-c288(w71) -> ()  [unwired: 1 out]
      n736 = Build Array(w66, w66, w66, w66, w66, w66, w66, w66) -> (w67:i16[])
      n737 = xnode "Output Shut Down"("FPGA VI Reference In"=w74, "error in"=w73, "AO"=w67, "INHB X"=w68, "INHB Y"=w68, "INHB Z"=w68, "INHB OCT Mot"=w68) -> ("FPGA VI Reference Out"=w82:refnum<k20>, "error out"=w81:errorcluster)
    }
    frame #3 {
      # "Reset Flags"
      n738 = disable-structure shown="Disabled" {
        disable-tunnel: w1062 -> [w1064 _]
        frame Disabled {
          n739 = Close File(refnum=w1064) -> ()  [unwired: 1 in, 2 out]
        }
        frame Enabled {
        }
      }
      n740 = disable-structure shown="Disabled" {
        disable-tunnel: w1058 -> [w1063 _]
        frame Disabled {
          n741 = UDP Close(connection ID=w1063) -> ()  [unwired: 1 in, 2 out]
        }
        frame Enabled {
        }
      }
      n742 = global write "Global Variables.vi" "irrigate"(FALSE ("irrigate")) -> ()
    }
    frame #4 {
      # "Close Application"
      n743 = xnode "FPGA Reset"("FPGA VI Reference In"=w1070, "error in"=w1069) -> ("FPGA VI Reference Out"=w1065:refnum<k20>, "error out"=w1066:errorcluster)
      n744 = global read "Global Variables.vi" "armID"() -> (w1068:i32)
      n745 = dll-call lib="D:/Kevin/IRISS V2 dev/Host Demo/Functions/EyeRobotDLL.dll" fn="CloseRobot" label="Close"("id"=w1068) -> ()  [unwired: 5 in, 2 out]
      n746 = xnode "Close FPGA VI Reference"("FPGA VI Reference In"=w1065, "error in"=w1066) -> ("error out"=→"Error(s) Out on Program End":errorcluster)
    }
  }
